vi "HEWH MW100.vi"(8 "error in":errorcluster, 11 "Message Queues out":T3) -> (0 "error out":errorcluster)   [LabVIEW 2023]
uses:
  Tenney/support/Message Queue/All Message Queues.ctl
  Tenney/support/Message Queue/Message Cluster.ctl
  Type Definitions/HEWH MW100 Data Cluster.ctl
  Custom Instrument Control/MW100/Type Definitions/HEWH Module 4 Relay Status.ctl
  Custom Instrument Control/MW100/Type Definitions/HEWH MW100 Channel Numbers.ctl
  Type Definitions/HEWH Normally Open Valve Control.ctl
  Type Definitions/HEWH Valve Bank Positions.ctl
  Type Definitions/HEWH Normally Closed Valve Control.ctl
  FVIR and LDO/support/Message Queue/Enqueue Message (Single).vi
  <vilib>/NI/Modbus Library/API/Wrapper/Create TCP Master.vi
  <vilib>/NI/Modbus Library/API/Master/Modbus Master.lvclass
  FVIR and LDO/support/Message Queue/Message Queue.lvlib
  Custom Instrument Control/MW100/Type Definitions/Station ID Selector.ctl
  Custom Instrument Control/Intellifaucet/Type Definitions/INTELLIFAUCET Set Mode.ctl
  <vilib>/NI/Modbus Library/API/Wrapper/API Main.lvlib
  Tenney/support/Message Queue/Tenney Message Queue.lvlib
panel:
  out "Loop Count":i32
  in  "Use Micro Amp Set":bool
  out "MW100 Data":T1
  in  "Pressurize Tank?":bool=TRUE
  in  "Debug":bool
  out "Debug":string[](array[string])
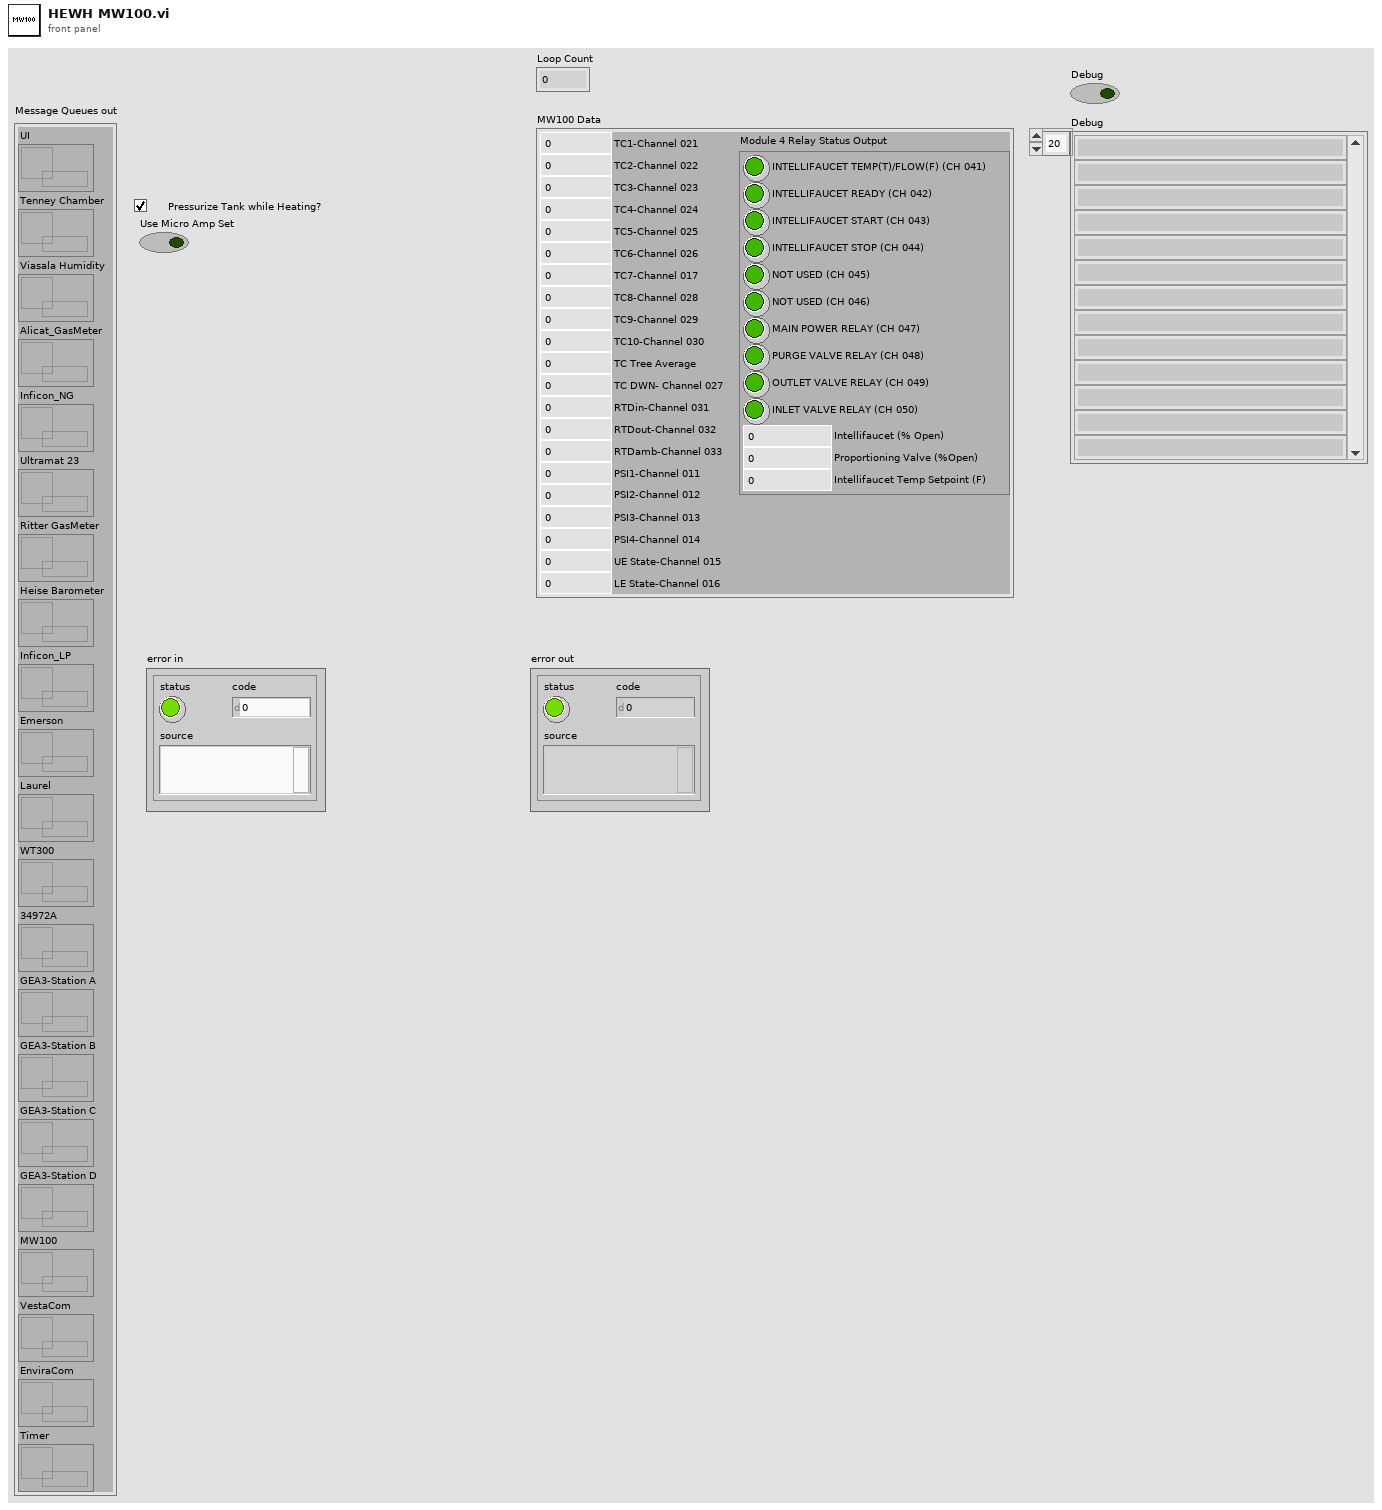
[diagram p1: front panel]
types:
  T1 = typedef "HEWH MW100 Data Cluster.ctl" = cluster{"TC1-Channel 021":dbl, "TC2-Channel 022":dbl, "TC3-Channel 023":dbl, "TC4-Channel 024":dbl, "TC5-Channel 025":dbl, "TC6-Channel 026":dbl, "TC7-Channel 017":dbl, "TC8-Channel 028":dbl, "TC9-Channel 029":dbl, "TC10-Channel 030":dbl, "TC Tree Average":dbl, "TC DWN- Channel 027":dbl, "RTDin-Channel 031":dbl, "RTDout-Channel 032":dbl, "RTDamb-Channel 033":dbl, "PSI1-Channel 011":dbl, "PSI2-Channel 012":dbl, "PSI3-Channel 013":dbl, "PSI4-Channel 014":dbl, "UE State-Channel 015":dbl, "LE State-Channel 016":dbl, "Module 4 Relay Status Output":T2}
  T2 = typedef "HEWH Module 4 Relay Status.ctl" = cluster{"INTELLIFAUCET TEMP(T)/FLOW(F) (CH 041)":bool, "INTELLIFAUCET READY (CH 042)":bool, "INTELLIFAUCET START (CH 043)":bool, "INTELLIFAUCET STOP (CH 044)":bool, "MAIN POWER RELAY (CH 047)":bool, "NOT USED (CH 045)":bool, "NOT USED (CH 046)":bool, "PURGE VALVE RELAY (CH 048)":bool, "OUTLET VALVE RELAY (CH 049)":bool, "INLET VALVE RELAY (CH 050)":bool, "Intellifaucet (% Open)":dbl, "Proportioning Valve (%Open)":dbl, "Intellifaucet Temp Setpoint (F)":dbl}
  T3 = typedef "Tenney Message Queue.lvlib/All Message Queues.ctl" = cluster{"UI":refnum<queue>, "Tenney Chamber":refnum<queue>, "Viasala Humidity":refnum<queue>, "Alicat_GasMeter":refnum<queue>, "Inficon_NG":refnum<queue>, "Ultramat 23":refnum<queue>, "Ritter GasMeter":refnum<queue>, "Heise Barometer":refnum<queue>, "Inficon_LP":refnum<queue>, "Emerson":refnum<queue>, "Laurel":refnum<queue>, "WT300":refnum<queue>, "34972A":refnum<queue>, "GEA3-Station A":refnum<queue>, "GEA3-Station B":refnum<queue>, "GEA3-Station C":refnum<queue>, "GEA3-Station D":refnum<queue>, "MW100":refnum<queue>, "VestaCom":refnum<queue>, "EnviraCom":refnum<queue>, "Timer":refnum<queue>}
  T4 = typedef "HEWH MW100 Channel Numbers.ctl" = string
  T5 = typedef "HEWH Normally Open Valve Control.ctl" = string
  T6 = typedef "HEWH Valve Bank Positions.ctl" = enum16{"Heating", "Purge", "Resting", "Draw"}
  T7 = typedef "HEWH Normally Closed Valve Control.ctl" = string
  T8 = typedef "Station ID Selector.ctl" = enum16{"", "A", "B", "C", "D", "Global"}
  T9 = typedef "INTELLIFAUCET Set Mode.ctl" = enum16{"Adjust Temp", "Adjust Flow", "Start Flow", "Stop Flow", "Hold Start", "Hold Stop", "Release Start", "Release Stop", "Temp/Flow Relay", "Adjust Prop Valve"}
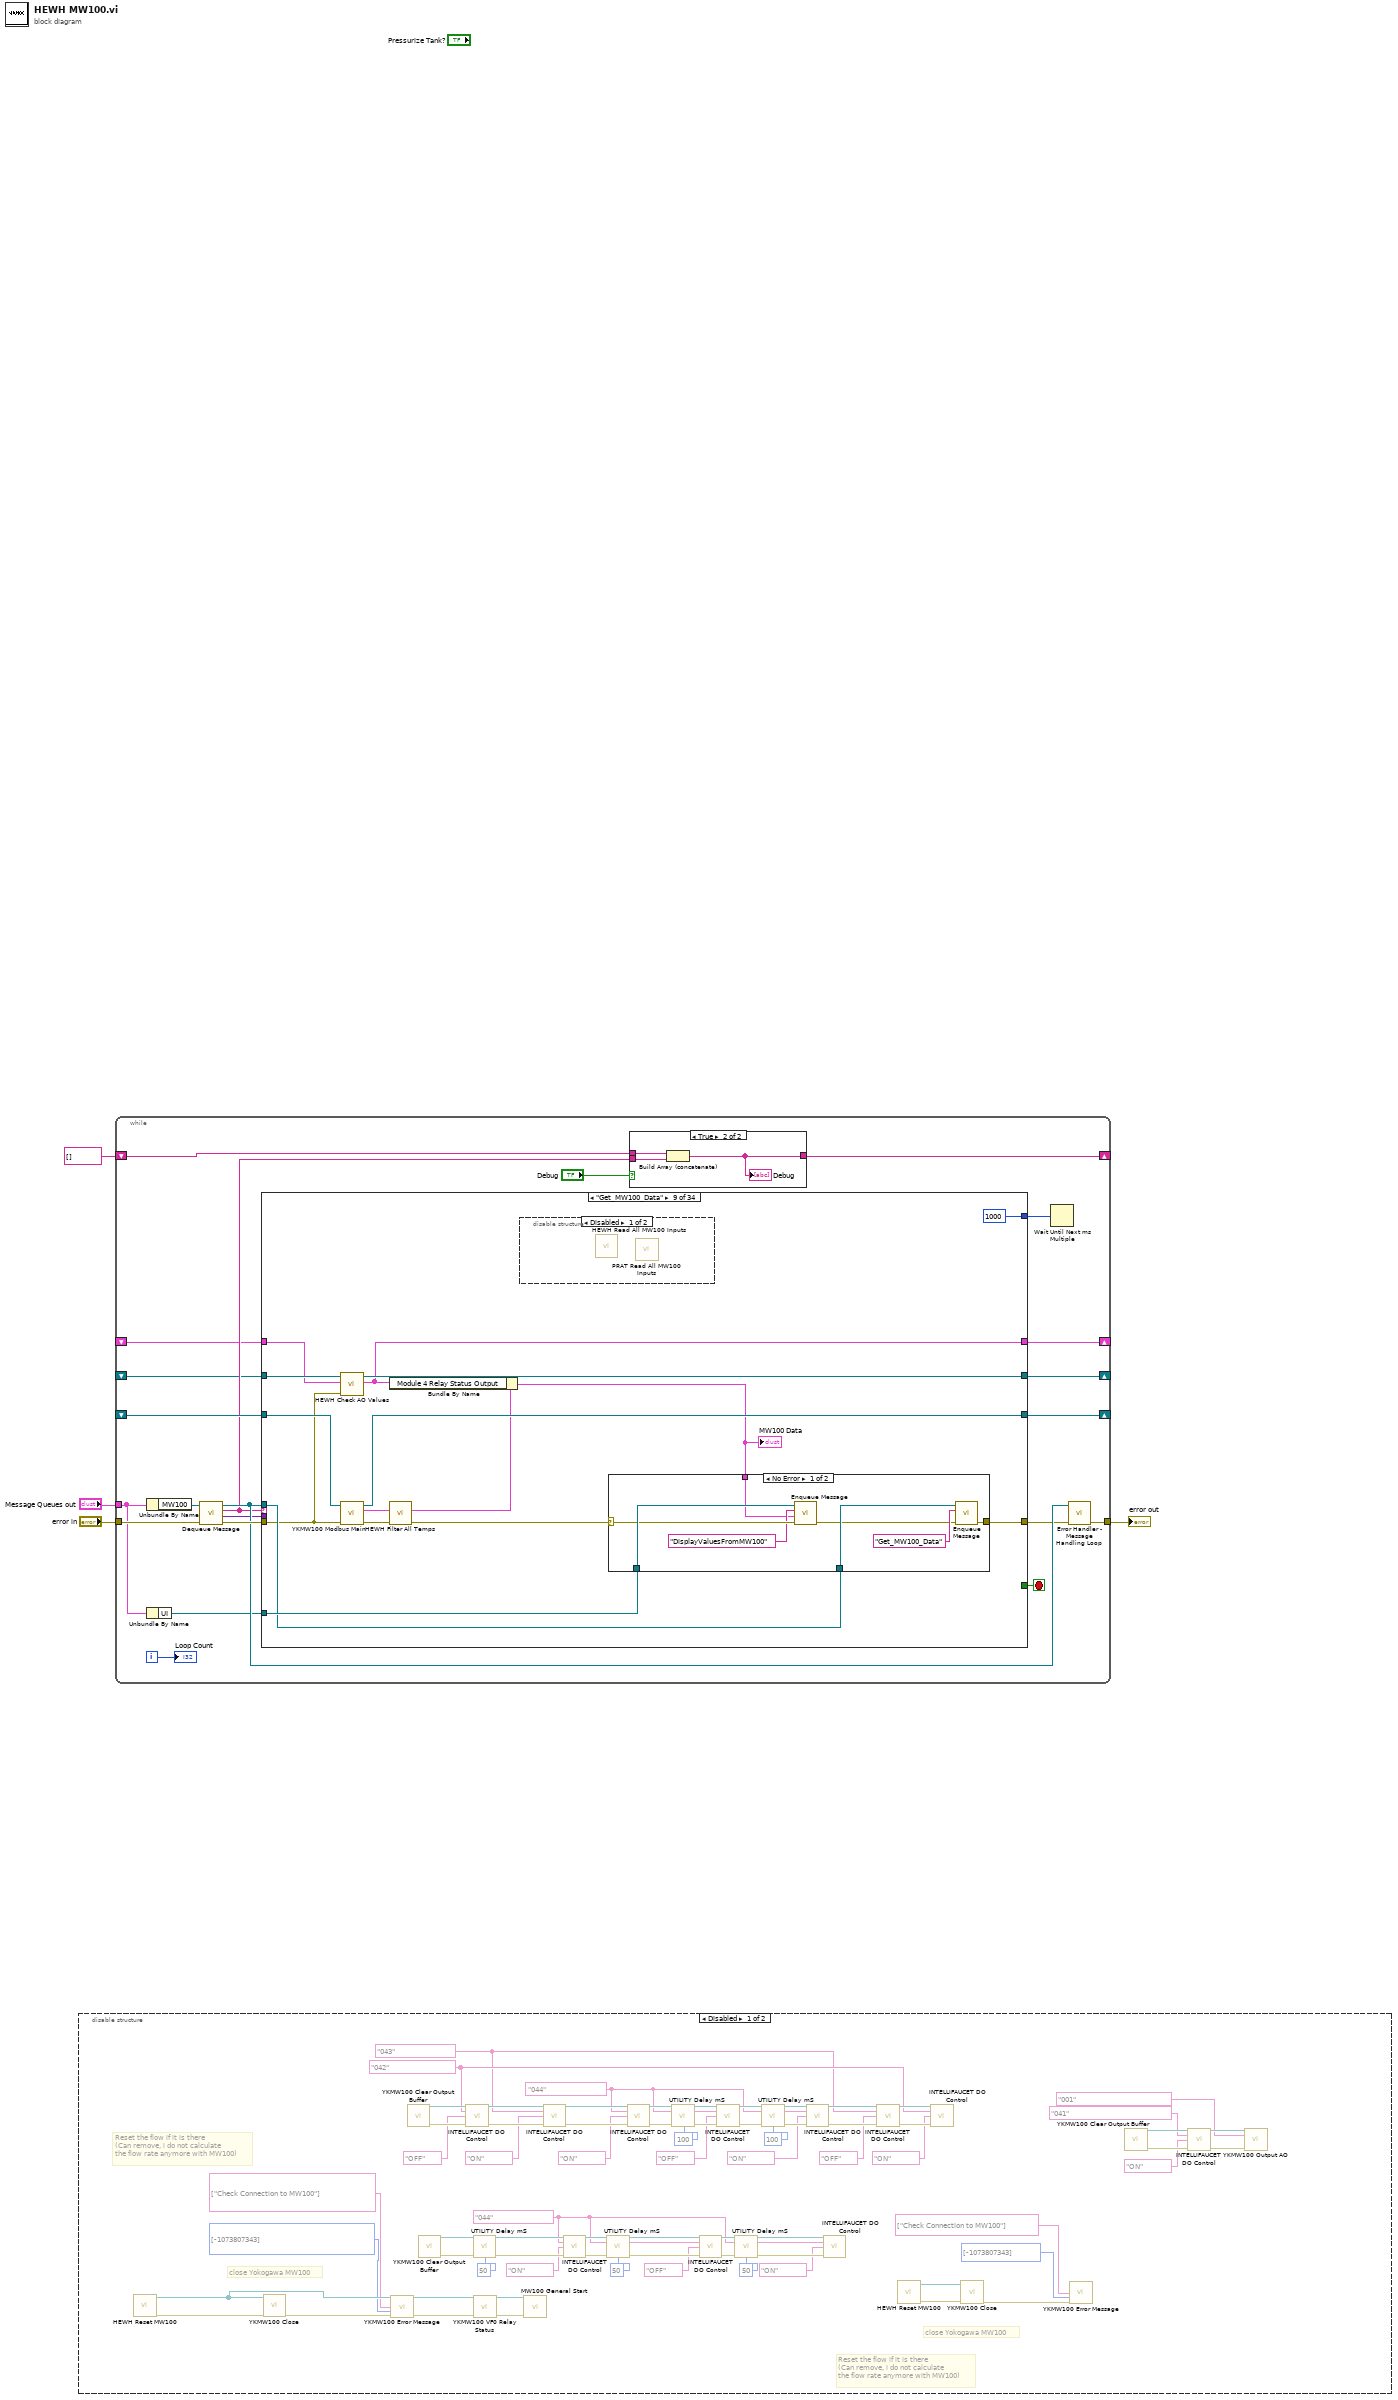
[diagram p0: block diagram]
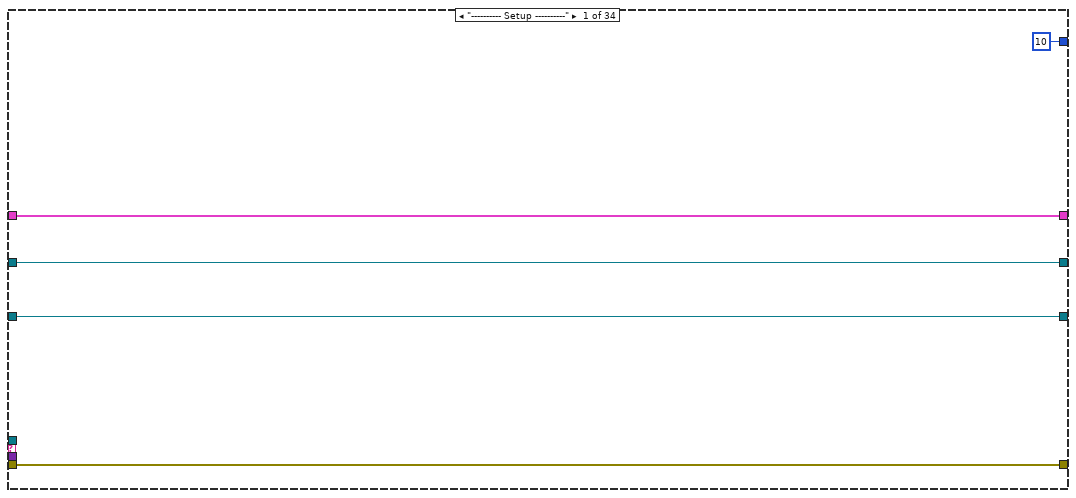
[diagram p4: hidden frame]
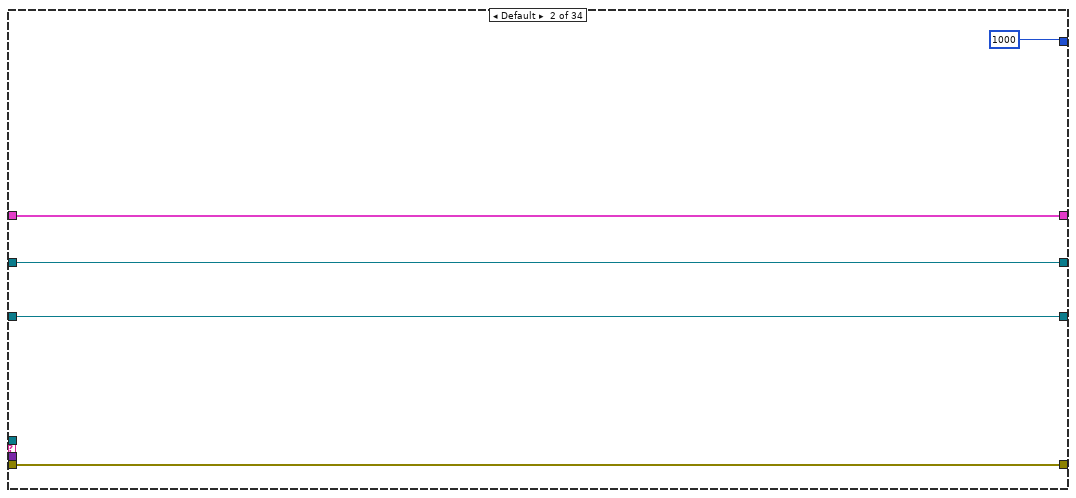
[diagram p5: hidden frame]
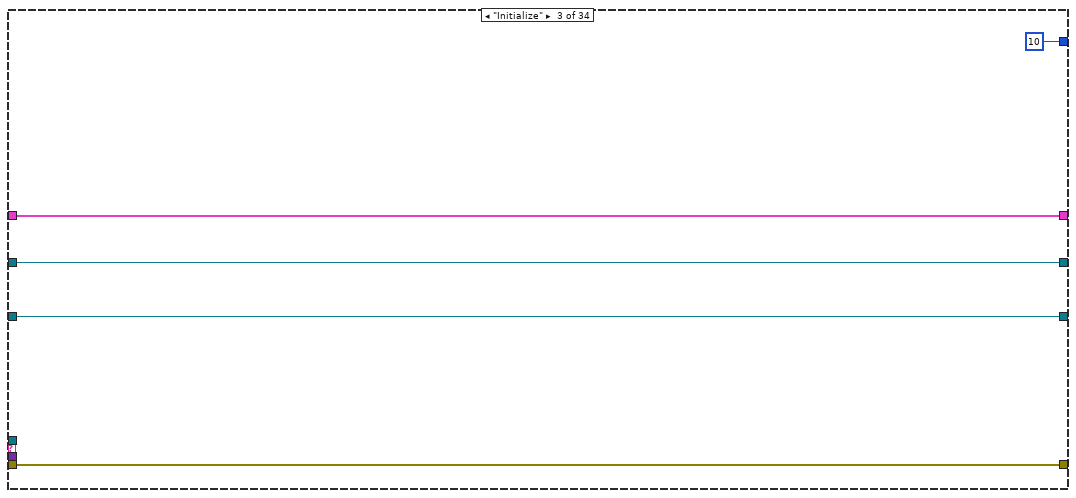
[diagram p6: hidden frame]
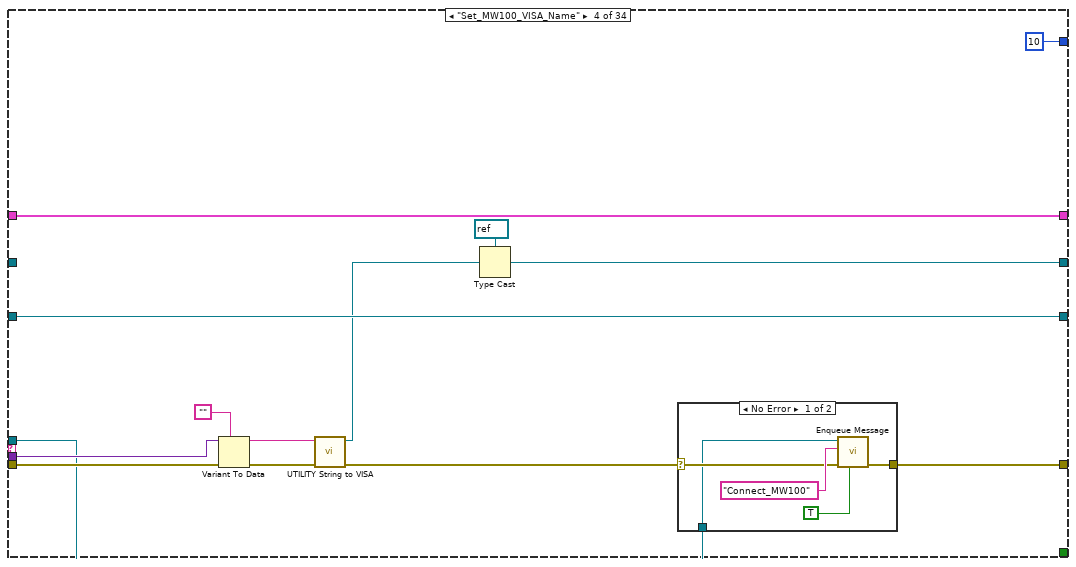
[diagram p7: hidden frame]
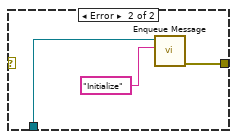
[diagram p8: hidden frame]
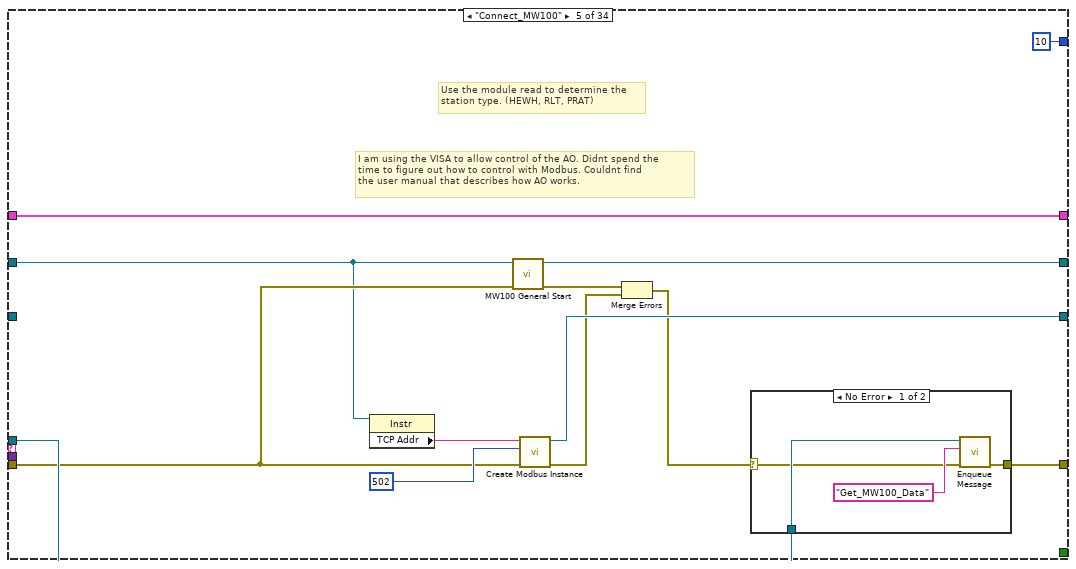
[diagram p9: hidden frame]
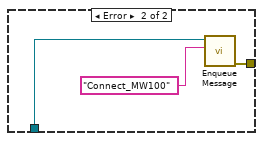
[diagram p10: hidden frame]
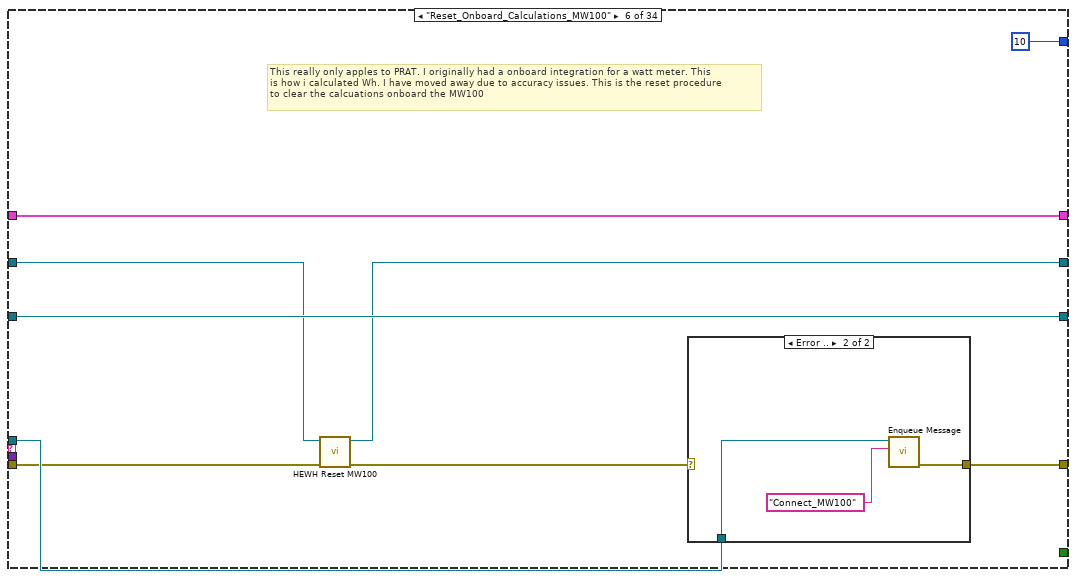
[diagram p11: hidden frame]
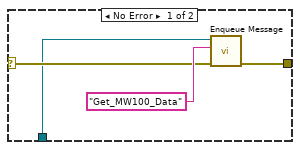
[diagram p12: hidden frame]
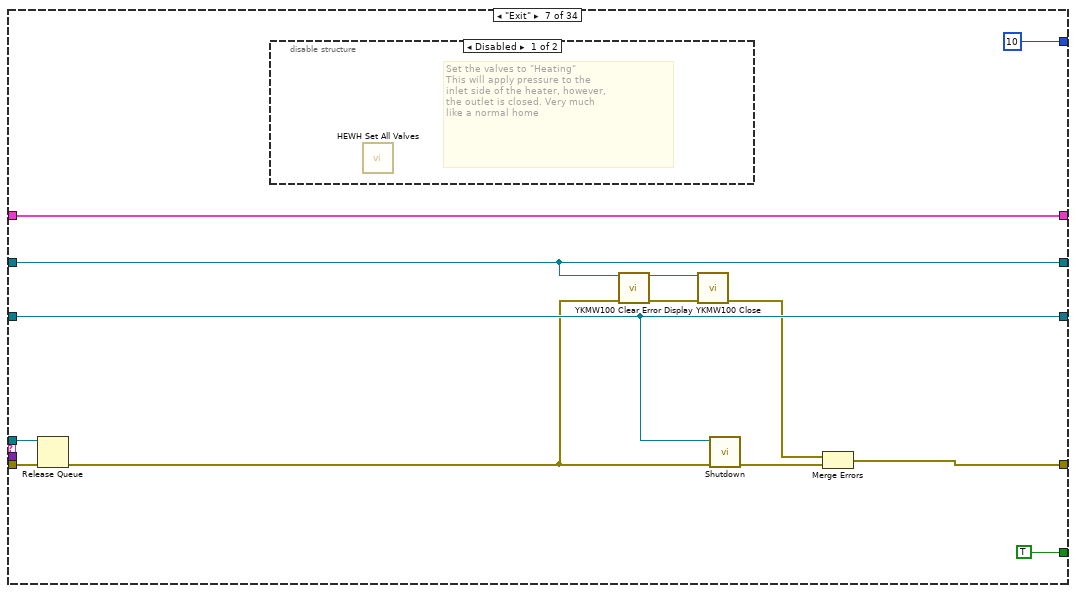
[diagram p13: hidden frame]
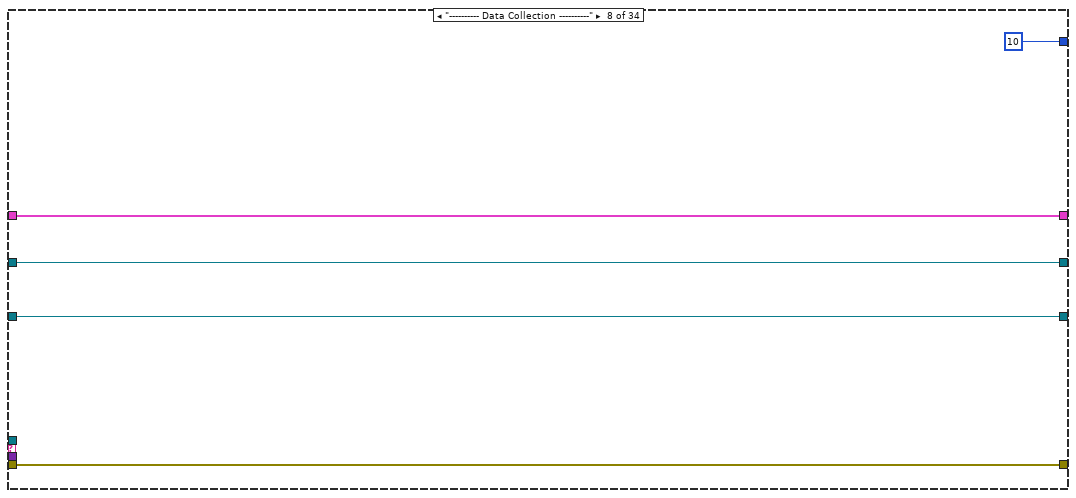
[diagram p15: hidden frame]
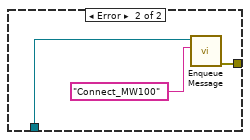
[diagram p17: hidden frame]
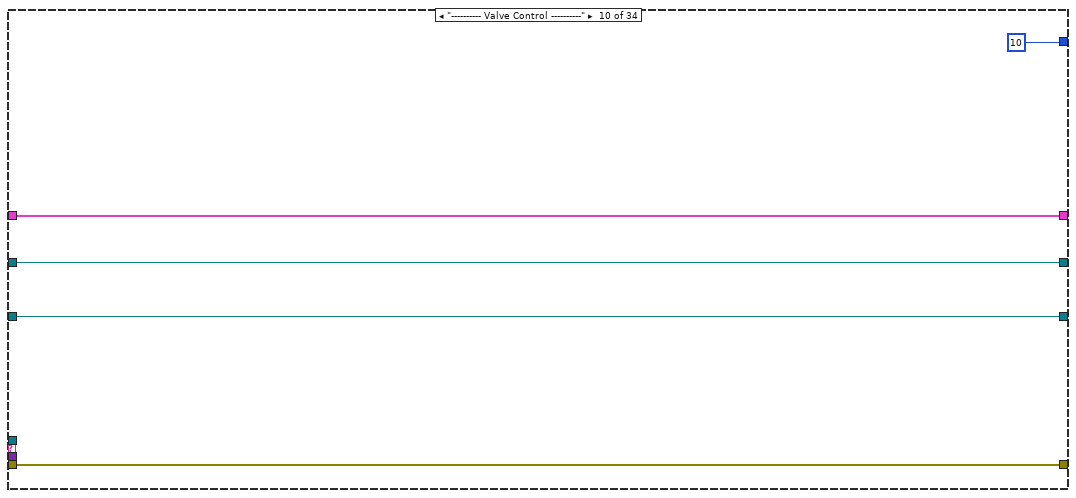
[diagram p18: hidden frame]
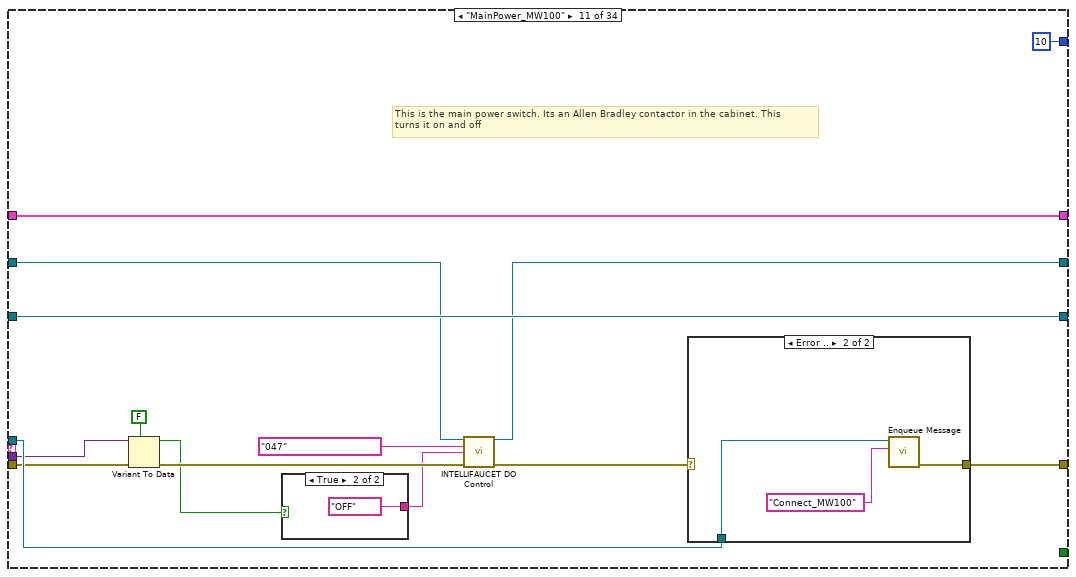
[diagram p19: hidden frame]
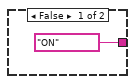
[diagram p20: hidden frame]
diagram:
  n1 = disable-structure shown="Disabled" {
    frame Disabled {
      w23 = T4 "042" ("HEWH MW100 Channel Numbers")
      w17 = T4 "043" ("HEWH MW100 Channel Numbers")
      w19 = T4 "044" ("HEWH MW100 Channel Numbers")
      w45 = T4 "044" ("HEWH MW100 Channel Numbers")
      # "Reset the flow if it is there\n(Can remove, i do not calculate\nthe flow rate anymore with MW100)"
      # "close Yokogawa MW100"
      # "Reset the flow if it is there\n(Can remove, i do not calculate\nthe flow rate anymore with MW100)"
      # "close Yokogawa MW100"
      n2 = call "HEWH Reset MW100.vi"() -> ("error out"=w64:errorcluster, "MW100 VISA Out"=w65:refnum<visa-resource-name>)  [unwired: 10 in]
      n3 = call "YKMW100 Close.vi"("VISA session"=w65, "error in (no error)"=w64) -> ("error out"=w63:errorcluster)  [unwired: 13 in]
      n4 = call "YKMW100 Error Message.vi"("VISA session"=w65, "User-Defined Descriptions"=string[] ["Check Connection to MW100"], "User-Defined Codes"=i32[] [-1073807343], "error in (no error)"=w63) -> ("dup VISA session"=w69:refnum<visa-resource-name>, "error out"=w68:errorcluster)  [unwired: 7 in, 3 out]
      n5 = call "YKMW100 Clear Output Buffer.vi"() -> ("dup VISA session"=w28:refnum<visa-resource-name>, "error out"=w29:errorcluster)  [unwired: 14 in]
      n6 = call "YKMW100 Clear Output Buffer.vi"() -> ("dup VISA session"=w52:refnum<visa-resource-name>, "error out"=w51:errorcluster)  [unwired: 14 in]
      n7 = call "INTELLIFAUCET DO Control.vi"("VISA session"=w28, "HEWH MW100 Channel Numbers"=w23, "Normally Open"=T5 "OFF", "Error In"=w29) -> ("dup VISA session"=w27:refnum<visa-resource-name>, "error out"=w26:errorcluster)  [unwired: 10 in]
      n8 = call "UTILITY Delay mS.vi"("Error In"=w51, "milliseconds to wait"=u32 50) -> ("Error Out"=w50:errorcluster)  [unwired: 13 in]
      n9 = call "YKMW100 VF0 Relay Status.vi"("MW100"=w69, "Error In"=w68) -> ("MW100 Out"=w66:refnum<visa-resource-name>, "error out"=w67:errorcluster)  [unwired: 9 in, 3 out]
      n10 = call "MW100 General Start.vi"("error in (no error)"=w67, "MW100 Input"=w66) -> ()  [unwired: 8 in, 2 out]
      n11 = call "INTELLIFAUCET DO Control.vi"("VISA session"=w27, "HEWH MW100 Channel Numbers"=w17, "Normally Open"=T5 "ON", "Error In"=w26) -> ("dup VISA session"=w35:refnum<visa-resource-name>, "error out"=w36:errorcluster)  [unwired: 10 in]
      n12 = call "INTELLIFAUCET DO Control.vi"("VISA session"=w52, "HEWH MW100 Channel Numbers"=w45, "Normally Open"=T5 "ON" ("Normally Open Valve"), "Error In"=w50) -> ("dup VISA session"=w53:refnum<visa-resource-name>, "error out"=w55:errorcluster)  [unwired: 10 in]
      n13 = call "UTILITY Delay mS.vi"("Error In"=w55, "milliseconds to wait"=u32 50) -> ("Error Out"=w54:errorcluster)  [unwired: 13 in]
      n14 = call "INTELLIFAUCET DO Control.vi"("VISA session"=w35, "HEWH MW100 Channel Numbers"=w19, "Normally Open"=T5 "ON" ("Normally Open Valve"), "Error In"=w36) -> ("dup VISA session"=w39:refnum<visa-resource-name>, "error out"=w38:errorcluster)  [unwired: 10 in]
      n15 = call "UTILITY Delay mS.vi"("Error In"=w38, "milliseconds to wait"=u32 100) -> ("Error Out"=w37:errorcluster)  [unwired: 13 in]
      n16 = call "INTELLIFAUCET DO Control.vi"("VISA session"=w53, "HEWH MW100 Channel Numbers"=w45, "Normally Open"=T5 "OFF" ("Normally Open Valve"), "Error In"=w54) -> ("dup VISA session"=w49:refnum<visa-resource-name>, "error out"=w48:errorcluster)  [unwired: 10 in]
      n17 = call "INTELLIFAUCET DO Control.vi"("VISA session"=w39, "HEWH MW100 Channel Numbers"=w19, "Normally Open"=T5 "OFF", "Error In"=w37) -> ("dup VISA session"=w33:refnum<visa-resource-name>, "error out"=w31:errorcluster)  [unwired: 10 in]
      n18 = call "UTILITY Delay mS.vi"("Error In"=w48, "milliseconds to wait"=u32 50) -> ("Error Out"=w47:errorcluster)  [unwired: 13 in]
      n19 = call "UTILITY Delay mS.vi"("Error In"=w31, "milliseconds to wait"=u32 100) -> ("Error Out"=w30:errorcluster)  [unwired: 13 in]
      n20 = call "INTELLIFAUCET DO Control.vi"("VISA session"=w33, "HEWH MW100 Channel Numbers"=w19, "Normally Open"=T5 "ON", "Error In"=w30) -> ("dup VISA session"=w32:refnum<visa-resource-name>, "error out"=w34:errorcluster)  [unwired: 10 in]
      n21 = call "INTELLIFAUCET DO Control.vi"("VISA session"=w49, "HEWH MW100 Channel Numbers"=w45, "Normally Open"=T5 "ON" ("Normally Open Valve"), "Error In"=w47) -> ()  [unwired: 10 in, 2 out]
      n22 = call "INTELLIFAUCET DO Control.vi"("VISA session"=w32, "HEWH MW100 Channel Numbers"=w17, "Normally Open"=T5 "OFF" ("Normally Open Valve"), "Error In"=w34) -> ("dup VISA session"=w25:refnum<visa-resource-name>, "error out"=w24:errorcluster)  [unwired: 10 in]
      n23 = call "HEWH Reset MW100.vi"() -> ("error out"=w59:errorcluster, "MW100 VISA Out"=w60:refnum<visa-resource-name>)  [unwired: 10 in]
      n24 = call "INTELLIFAUCET DO Control.vi"("VISA session"=w25, "HEWH MW100 Channel Numbers"=w23, "Normally Open"=T5 "ON", "Error In"=w24) -> ()  [unwired: 10 in, 2 out]
      n25 = call "YKMW100 Close.vi"("VISA session"=w60, "error in (no error)"=w59) -> ("error out"=w58:errorcluster)  [unwired: 13 in]
      n26 = call "YKMW100 Error Message.vi"("User-Defined Descriptions"=string[] ["Check Connection to MW100"], "User-Defined Codes"=i32[] [-1073807343], "error in (no error)"=w58) -> ()  [unwired: 8 in, 5 out]
      n27 = call "YKMW100 Clear Output Buffer.vi"() -> ("dup VISA session"=w10:refnum<visa-resource-name>, "error out"=w11:errorcluster)  [unwired: 14 in]
      n28 = call "INTELLIFAUCET DO Control.vi"("VISA session"=w10, "HEWH MW100 Channel Numbers"=T4 "041", "Normally Open"=T5 "ON" ("Normally Open Valve"), "Error In"=w11) -> ("dup VISA session"=w9:refnum<visa-resource-name>, "error out"=w8:errorcluster)  [unwired: 10 in]
      n29 = call "YKMW100 Output AO.vi"("VISA session"=w9, "Channel String (001)"=T4 "001" ("HEWH MW100 Channel Numbers"), "error in (no error)"=w8) -> ()  [unwired: 11 in, 2 out]
    }
    frame Enabled {
    }
  }
  n30 = while {
    tunnel: "Message Queues out" -> [w82]
    tunnel: "error in" -> [w90]
    tunnel: [w86] -> w3
    shift-right: [w84] -> _
    shift-left: _ -> [w83]
    shift-right: [w78] -> _
    shift-left: string[] [] -> [w79]
    shift-right: [w75] -> _
    shift-left: _ -> [w74]
    shift-right: [w71] -> _
    shift-left: _ -> [w70]
    i -> [w73]
    stop <- w88 stop-if-true
    n31 = Unbundle By Name(w82) -> ("MW100"=w91:refnum<queue>)
    n32 = Unbundle By Name(w82) -> ("UI"=w81:refnum<queue>)
    n33 = call "Dequeue Message.vi"("error in (no error)"=w90, "Message Queue"=w91) -> ("error out"=w89:errorcluster, "Message Data"=w76:variant, "Message"=w80:string, "dup Message Queue"=w87:refnum<queue>)  [unwired: 6 in]
    n34 = case shown="\"Get_MW100_Data\"" w80 {
      tunnel: w89 -> [w100 w103 w106 w119 w141 w157 w179 w186 w196 w218 w230 w252 w328 w404 w480 w557 w580 w604 w627 w650 w671 w692 w713 w734 w755 w776 w797 w812 w818 w835 w861 w888 w905 w923]
      tunnel: [w100 w103 w106 w121 w145 w161 w176 w186 w201 w218 w233 w255 w331 w407 w483 w560 w583 w607 w630 w653 w674 w695 w716 w737 w758 w779 w800 w812 w822 w840 w864 w890 w905 w925] -> w85
      tunnel: [_ _ _ _ _ _ TRUE _ _ _ _ _ _ _ _ _ _ _ _ _ _ _ _ _ _ _ _ _ _ _ _ _ _ _] -> w88
      tunnel: w87 -> [_ _ _ w111 w144 w160 w180 _ w200 _ w232 w254 w330 w406 w482 w559 w582 w606 w629 w652 w673 w694 w715 w736 w757 w778 w799 _ w821 w839 w863 w889 _ w924]
      tunnel: [w99 w105 w110 w124 w142 w158 w178 w185 w198 w217 w231 w253 w329 w405 w481 w558 w581 w605 w628 w651 w672 w693 w714 w735 w756 w777 w798 w811 w820 w838 w862 w886 w904 w921] -> w84
      tunnel: w83 -> [w99 w105 w110 w124 _ w158 w178 w185 w199 w217 w231 w253 w329 w405 w481 w558 w581 w605 w628 w651 w672 w693 w714 w735 w756 w777 w798 w811 w820 w838 w862 w886 w904 w921]
      tunnel: w81 -> [_ _ _ _ _ _ _ _ w202 _ _ _ _ _ _ _ _ _ _ _ _ _ _ _ _ _ _ _ _ _ _ _ _ _]
      tunnel: w76 -> [_ _ _ w116 _ _ _ _ _ _ w229 w251 w327 w403 w479 w556 w579 w603 w626 w649 w670 w691 w712 w733 w754 w775 w796 _ _ _ w860 w887 _ w922]
      tunnel: [w98 w104 w109 w112 w140 w155 w172 w184 w191 w216 w223 w245 w322 w398 w474 w551 w574 w598 w621 w647 w665 w687 w708 w728 w750 w771 w791 w810 w816 w832 w852 w880 w903 w909] -> w75
      tunnel: w74 -> [w98 w104 w109 _ w133 w156 w172 w184 w197 w216 w224 w246 w323 w399 w475 w553 w575 w599 w622 w648 w666 w688 w709 w729 w751 w772 w792 w810 w819 w833 w851 w883 w903 w915]
      tunnel: [u32 10 ("millisecond multiple") u32 1000 ("millisecond multiple") u32 10 ("millisecond multiple") u32 10 ("millisecond multiple") u32 10 ("millisecond multiple") u32 10 ("millisecond multiple") u32 10 ("millisecond multiple") u32 10 ("millisecond multiple") u32 1000 ("millisecond multiple") u32 10 ("millisecond multiple") u32 10 ("millisecond multiple") u32 10 ("millisecond multiple") u32 10 ("millisecond multiple") u32 10 ("millisecond multiple") u32 10 ("millisecond multiple") u32 10 ("millisecond multiple") u32 10 ("millisecond multiple") u32 10 ("millisecond multiple") u32 10 ("millisecond multiple") u32 10 ("millisecond multiple") u32 10 ("millisecond multiple") u32 10 ("millisecond multiple") u32 10 ("millisecond multiple") u32 10 ("millisecond multiple") u32 10 ("millisecond multiple") u32 10 ("millisecond multiple") u32 10 ("millisecond multiple") u32 10 ("millisecond multiple") u32 10 ("millisecond multiple") u32 10 ("millisecond multiple") u32 10 ("millisecond multiple") u32 10 ("millisecond multiple") u32 10 ("millisecond multiple") u32 10 ("millisecond multiple")] -> w72
      tunnel: [w96 w101 w107 w122 w134 w153 w169 w182 w188 w214 w219 w243 w319 w395 w471 w547 w570 w594 w617 w640 w661 w682 w703 w724 w745 w766 w787 w808 w813 w831 w849 w875 w901 w906] -> w71
      tunnel: w70 -> [w96 w101 w107 w122 w134 w153 w169 w182 w187 w214 w219 w243 w319 w395 w471 w547 w570 w594 w617 w640 w661 w682 w703 w724 w745 w766 w787 w808 w813 w831 w849 w875 w901 w906]
      frame "---------- Setup ----------" {
      }
      frame Default {
      }
      frame "Initialize" {
      }
      frame "Set_MW100_VISA_Name" {
        n35 = Variant To Data(error in=w119, type="", Variant=w116) -> (data=w115:string, error out=w118:errorcluster)
        n36 = call "UTILITY String to VISA.vi"("error in (no error)"=w118, "VISA Name"=w115) -> ("error out"=w117:errorcluster, "VISA resource name out"=w114:refnum<visa-resource-name>)  [unwired: 8 in]
        n37 = Type Cast(type=refnum<visa-resource-name> refnum ("dup VISA session"), x=w114) -> (*(type *) &x=w112:refnum<visa-resource-name>)
        n38 = case shown="No Error" w117 {
          selector: w117 -> [w126 _]
          tunnel: [w127 w131] -> w121
          tunnel: w111 -> [w125 w130]
          frame No Error {
            n39 = call-poly "Enqueue Message.vi"("Priority Message? (F)"=TRUE, "error in (no error)"=w126, "Message"="Connect_MW100", "Message Queue"=w125) -> ("error out"=w127:errorcluster)  [unwired: 6 in, 1 out]
          }
          frame Error {
            n40 = call-poly "Enqueue Message.vi"("Message"="Initialize", "Message Queue"=w130) -> ("error out"=w131:errorcluster)  [unwired: 8 in, 1 out]
          }
        }
      }
      frame "Connect_MW100" {
        # "Use the module read to determine the \nstation type. (HEWH, RLT, PRAT)"
        # "I am using the VISA to allow control of the AO. Didnt spend the \ntime to figure out how to control with Modbus. Couldnt find\nthe user manual that describes how AO works."
        n41 = property class="Instr"(reference=w133) -> ("TCP Addr"=w136:string)  [unwired: 1 in, 2 out]
        n42 = call "MW100 General Start.vi"("error in (no error)"=w141, "MW100 Input"=w133) -> ("error out"=w139:errorcluster, "MW100 Output"=w140:refnum<visa-resource-name>)  [unwired: 8 in]
        n43 = call-poly <vilib>:"Create Modbus Instance.vi"("error in"=w141, "port (502)"=u16 502, "address"=w136) -> ("error out"=w138:errorcluster, "TCP master instance"=w142:refnum<class "Modbus Master.lvclass">)  [unwired: 7 in]
        n44 = Merge Errors(w139, w138) -> (w137:errorcluster)
        n45 = case shown="No Error" w137 {
          selector: w137 -> [w146 _]
          tunnel: [w148 w151] -> w145
          tunnel: w144 -> [w147 w150]
          frame No Error {
            n46 = call-poly "Enqueue Message.vi"("error in (no error)"=w146, "Message"="Get_MW100_Data", "Message Queue"=w147) -> ("error out"=w148:errorcluster)  [unwired: 7 in, 1 out]
          }
          frame Error {
            n47 = call-poly "Enqueue Message.vi"("Message"="Connect_MW100", "Message Queue"=w150) -> ("error out"=w151:errorcluster)  [unwired: 8 in, 1 out]
          }
        }
      }
      frame "Reset_Onboard_Calculations_MW100" {
        # "This really only apples to PRAT. I originally had a onboard integration for a watt meter. This \nis how i calculated Wh. I have moved away due to accuracy issues. This is the reset procedure\nto clear the calcuations onboard the MW100"
        n48 = call "HEWH Reset MW100.vi"("error in (no error)"=w157, "MW100 VISA In"=w156) -> ("error out"=w159:errorcluster, "MW100 VISA Out"=w155:refnum<visa-resource-name>)  [unwired: 8 in]
        n49 = case shown="Error .." w159 {
          selector: w159 -> [w164 _]
          tunnel: [w163 w167] -> w161
          tunnel: w160 -> [w162 w166]
          frame No Error {
            n50 = call-poly "Enqueue Message.vi"("error in (no error)"=w164, "Message"="Get_MW100_Data", "Message Queue"=w162) -> ("error out"=w163:errorcluster)  [unwired: 7 in, 1 out]
          }
          frame Error {
            n51 = call-poly "Enqueue Message.vi"("Message"="Connect_MW100", "Message Queue"=w166) -> ("error out"=w167:errorcluster)  [unwired: 8 in, 1 out]
          }
        }
      }
      frame "Exit" {
        n52 = Release Queue(queue=w180, error in (no error)=w179) -> (error out=w174:errorcluster)  [unwired: 1 in, 2 out]
        n53 = disable-structure shown="Disabled" {
          frame Disabled {
            # "Set the valves to \"Heating\"\nThis will apply pressure to the\ninlet side of the heater, however,\nthe outlet is closed. Very much\nlike a normal home"
            n54 = call "HEWH Set All Valves.vi"() -> ()  [unwired: 10 in, 2 out]
          }
          frame Enabled {
          }
        }
        n55 = call "YKMW100 Clear Error Display.vi"("VISA session"=w172, "error in (no error)"=w174) -> ("dup VISA session"=w173:refnum<visa-resource-name>, "error out"=w175:errorcluster)  [unwired: 10 in, 2 out]
        n56 = call "YKMW100 Close.vi"("VISA session"=w173, "error in (no error)"=w175) -> ("error out"=w171:errorcluster)  [unwired: 13 in]
        n57 = call-dynamic "Shutdown.vi"("error in"=w174, "Modbus master in"=w178) -> ("error out"=w177:errorcluster)  [unwired: 9 in]
        n58 = Merge Errors(w171, w177) -> (w176:errorcluster)
      }
      frame "---------- Data Collection ----------" {
      }
      frame "Get_MW100_Data" {
        n59 = call "HEWH Check AO Values.vi"("error in (no error)"=w196, "Module 4 Relay Status Input"=w187, "VISA session"=w197) -> ("Module 4 Relay Status Output"=w188:T2, "dup VISA session"=w191:refnum<visa-resource-name>)  [unwired: 6 in, 1 out]
        n60 = call "YKMW100 Modbus Main.vi"("error in (no error)"=w196, "Modbus master in"=w199) -> ("error out"=w195:errorcluster, "MW Output"=w194:T1, "Modbus master out"=w198:refnum<class "Modbus Master.lvclass">)  [unwired: 7 in]
        n61 = call "HEWH Filter All Temps.vi"("error in (no error)"=w195, "Pressure Adjusted in"=w194) -> ("error out"=w189:errorcluster, "Pressure Adjusted out"=w193:T1)  [unwired: 7 in, 1 out]
        n62 = Bundle By Name(cluster=w193, "Module 4 Relay Status Output"=w188) -> (w192:T1)
        "MW100 Data" <- w192
        n63 = disable-structure shown="Disabled" {
          frame Disabled {
            n64 = call "HEWH Read All MW100 Inputs.vi"() -> ()  [unwired: 14 in, 2 out]
            n65 = call "PRAT Read All MW100 Inputs.vi"() -> ()  [unwired: 12 in, 4 out]
          }
          frame Enabled {
          }
        }
        n66 = case shown="No Error" w189 {
          selector: w189 -> [w205 _]
          tunnel: w202 -> [w210 _]
          tunnel: [w209 w212] -> w201
          tunnel: w200 -> [w208 w211]
          tunnel: w192 -> [w203 _]
          frame No Error {
            n67 = call-poly "Enqueue Message.vi"("error in (no error)"=w205, "Message Data"=w203, "Message"="DisplayValuesFromMW100", "Message Queue"=w210) -> ("error out"=w206:errorcluster)  [unwired: 6 in, 1 out]
            n68 = call-poly "Enqueue Message.vi"("error in (no error)"=w206, "Message"="Get_MW100_Data", "Message Queue"=w208) -> ("error out"=w209:errorcluster)  [unwired: 7 in, 1 out]
          }
          frame Error {
            n69 = call-poly "Enqueue Message.vi"("Message"="Connect_MW100", "Message Queue"=w211) -> ("error out"=w212:errorcluster)  [unwired: 8 in, 1 out]
          }
        }
      }
      frame "---------- Valve Control ----------" {
      }
      frame "MainPower_MW100" {
        # "This is the main power switch. Its an Allen Bradley contactor in the cabinet. This \nturns it on and off"
        n70 = Variant To Data(error in=w230, type=FALSE, Variant=w229) -> (data=w222:bool, error out=w227:errorcluster)
        n71 = case shown="True" w222 {
          tunnel: [T5 "ON" ("Normally Open Valve") T5 "OFF" ("Normally Open Valve")] -> w221
          frame False {
          }
          frame True {
          }
        }
        n72 = call "INTELLIFAUCET DO Control.vi"("VISA session"=w224, "HEWH MW100 Channel Numbers"=T4 "047", "Normally Open"=w221, "Error In"=w227) -> ("dup VISA session"=w223:refnum<visa-resource-name>, "error out"=w226:errorcluster)  [unwired: 10 in]
        n73 = case shown="Error .." w226 {
          selector: w226 -> [w238 _]
          tunnel: [w237 w241] -> w233
          tunnel: w232 -> [w236 w240]
          frame No Error {
            n74 = call-poly "Enqueue Message.vi"("error in (no error)"=w238, "Message"="Get_MW100_Data", "Message Queue"=w236) -> ("error out"=w237:errorcluster)  [unwired: 7 in, 1 out]
          }
          frame Error {
            n75 = call-poly "Enqueue Message.vi"("Message"="Connect_MW100", "Message Queue"=w240) -> ("error out"=w241:errorcluster)  [unwired: 8 in, 1 out]
          }
        }
      }
      frame "Set_Valves_StationA_MW100" {
        # "This is a function to actuate all of the valves to the proper position for heating,purge, resting, draw."
        n76 = disable-structure shown="Disabled" {
          frame Disabled {
            n77 = call "HEWH Solenoid Bank.vi"() -> ()  [unwired: 11 in, 5 out]
          }
          frame Enabled {
          }
        }
        n78 = Variant To Data(error in=w252, type=HEWH_Valve_Bank_Positions."Heating" ("Valve Bank Setting 2"), Variant=w251) -> (data=w249:T6, error out=w248:errorcluster)
        n79 = case shown="\"Heating\", Default" w249 {
          tunnel: w248 -> [w267 w279 w287 w305]
          tunnel: [w260 w274 w285 w298] -> w247
          tunnel: w246 -> [w259 w270 w284 w302]
          tunnel: [w256 w273 w286 w299] -> w245
          frame "Heating", Default {
            # "Check this one. Think its reversed."
            n80 = call "INTELLIFAUCET DO Control.vi"("VISA session"=w259, "HEWH MW100 Channel Numbers"=T4 "049", "Normally Open"=T5 "ON" ("Input Valve"), "Error In"=w267) -> ("dup VISA session"=w258:refnum<visa-resource-name>, "error out"=w264:errorcluster)  [unwired: 10 in]
            n81 = call "INTELLIFAUCET DO Control.vi"("VISA session"=w258, "HEWH MW100 Channel Numbers"=T4 "050", "Normally Open"=T5 "OFF" ("Input Valve"), "Error In"=w264) -> ("dup VISA session"=w257:refnum<visa-resource-name>, "error out"=w261:errorcluster)  [unwired: 10 in]
            n82 = call "HEWH_Normally_Closed_Solenoid.vi"("VISA session"=w257, "HEWH MW100 Channel Numbers"=T4 "048", "Normally Closed"=T7 "OFF" ("Normally Closed Valve"), "Error In"=w261) -> ("dup VISA session"=w256:refnum<visa-resource-name>, "error out"=w260:errorcluster)  [unwired: 10 in]
          }
          frame "Purge" {
            # "Check this one. Think its reversed."
            n83 = call "INTELLIFAUCET DO Control.vi"("VISA session"=w270, "HEWH MW100 Channel Numbers"=T4 "050", "Normally Open"=T5 "OFF" ("Input Valve"), "Error In"=w279) -> ("dup VISA session"=w272:refnum<visa-resource-name>, "error out"=w276:errorcluster)  [unwired: 10 in]
            n84 = call "INTELLIFAUCET DO Control.vi"("VISA session"=w272, "HEWH MW100 Channel Numbers"=T4 "049", "Normally Open"=T5 "ON" ("Input Valve"), "Error In"=w276) -> ("dup VISA session"=w271:refnum<visa-resource-name>, "error out"=w275:errorcluster)  [unwired: 10 in]
            n85 = call "HEWH_Normally_Closed_Solenoid.vi"("VISA session"=w271, "HEWH MW100 Channel Numbers"=T4 "048", "Normally Closed"=T7 "ON" ("Normally Closed Valve"), "Error In"=w275) -> ("dup VISA session"=w273:refnum<visa-resource-name>, "error out"=w274:errorcluster)  [unwired: 10 in]
          }
          frame "Resting" {
            # "Check this one. Think its reversed."
            n86 = call "INTELLIFAUCET DO Control.vi"("VISA session"=w284, "HEWH MW100 Channel Numbers"=T4 "050", "Normally Open"=T5 "ON" ("Input Valve"), "Error In"=w287) -> ("dup VISA session"=w295:refnum<visa-resource-name>, "error out"=w297:errorcluster)  [unwired: 10 in]
            n87 = call "INTELLIFAUCET DO Control.vi"("VISA session"=w295, "HEWH MW100 Channel Numbers"=T4 "049", "Normally Open"=T5 "OFF" ("Input Valve"), "Error In"=w297) -> ("dup VISA session"=w294:refnum<visa-resource-name>, "error out"=w296:errorcluster)  [unwired: 10 in]
            n88 = call "HEWH_Normally_Closed_Solenoid.vi"("VISA session"=w294, "HEWH MW100 Channel Numbers"=T4 "048", "Normally Closed"=T7 "OFF" ("Normally Closed Valve"), "Error In"=w296) -> ("dup VISA session"=w286:refnum<visa-resource-name>, "error out"=w285:errorcluster)  [unwired: 10 in]
          }
          frame "Draw" {
            # "Check this one. Think its reversed."
            n89 = call "HEWH_Normally_Closed_Solenoid.vi"("VISA session"=w302, "HEWH MW100 Channel Numbers"=T4 "048", "Normally Closed"=T7 "OFF" ("Normally Closed Valve"), "Error In"=w305) -> ("dup VISA session"=w301:refnum<visa-resource-name>, "error out"=w304:errorcluster)  [unwired: 10 in]
            n90 = call "INTELLIFAUCET DO Control.vi"("VISA session"=w301, "HEWH MW100 Channel Numbers"=T4 "050", "Normally Open"=T5 "OFF" ("Input Valve"), "Error In"=w304) -> ("dup VISA session"=w300:refnum<visa-resource-name>, "error out"=w303:errorcluster)  [unwired: 10 in]
            n91 = call "INTELLIFAUCET DO Control.vi"("VISA session"=w300, "HEWH MW100 Channel Numbers"=T4 "049", "Normally Open"=T5 "OFF" ("Input Valve"), "Error In"=w303) -> ("dup VISA session"=w299:refnum<visa-resource-name>, "error out"=w298:errorcluster)  [unwired: 10 in]
          }
        }
        n92 = case shown="Error .." w247 {
          selector: w247 -> [w314 _]
          tunnel: [w313 w317] -> w255
          tunnel: w254 -> [w312 w316]
          frame No Error {
            n93 = call-poly "Enqueue Message.vi"("error in (no error)"=w314, "Message"="Get_MW100_Data", "Message Queue"=w312) -> ("error out"=w313:errorcluster)  [unwired: 7 in, 1 out]
          }
          frame Error {
            n94 = call-poly "Enqueue Message.vi"("Message"="Connect_MW100", "Message Queue"=w316) -> ("error out"=w317:errorcluster)  [unwired: 8 in, 1 out]
          }
        }
      }
      frame "Set_Valves_StationB_MW100" {
        # "This is a function to actuate all of the valves to the proper position for heating,purge, resting, draw."
        n95 = Variant To Data(error in=w328, type=HEWH_Valve_Bank_Positions."Heating" ("Valve Bank Setting 2"), Variant=w327) -> (data=w324:T6, error out=w325:errorcluster)
        n96 = case shown="\"Draw\"" w324 {
          tunnel: w325 -> [w343 w355 w363 w381]
          tunnel: [w336 w350 w361 w374] -> w321
          tunnel: w323 -> [w335 w346 w360 w378]
          tunnel: [w332 w349 w362 w375] -> w322
          frame "Heating", Default {
            # "Check this one. Think its reversed."
            n97 = call "INTELLIFAUCET DO Control.vi"("VISA session"=w335, "HEWH MW100 Channel Numbers"=T4 "052", "Normally Open"=T5 "ON" ("Input Valve"), "Error In"=w343) -> ("dup VISA session"=w334:refnum<visa-resource-name>, "error out"=w340:errorcluster)  [unwired: 10 in]
            n98 = call "INTELLIFAUCET DO Control.vi"("VISA session"=w334, "HEWH MW100 Channel Numbers"=T4 "053", "Normally Open"=T5 "OFF" ("Input Valve"), "Error In"=w340) -> ("dup VISA session"=w333:refnum<visa-resource-name>, "error out"=w337:errorcluster)  [unwired: 10 in]
            n99 = call "HEWH_Normally_Closed_Solenoid.vi"("VISA session"=w333, "HEWH MW100 Channel Numbers"=T4 "051", "Normally Closed"=T7 "OFF" ("Normally Closed Valve"), "Error In"=w337) -> ("dup VISA session"=w332:refnum<visa-resource-name>, "error out"=w336:errorcluster)  [unwired: 10 in]
          }
          frame "Purge" {
            # "Check this one. Think its reversed."
            n100 = call "INTELLIFAUCET DO Control.vi"("VISA session"=w346, "HEWH MW100 Channel Numbers"=T4 "053", "Normally Open"=T5 "OFF" ("Input Valve"), "Error In"=w355) -> ("dup VISA session"=w348:refnum<visa-resource-name>, "error out"=w352:errorcluster)  [unwired: 10 in]
            n101 = call "INTELLIFAUCET DO Control.vi"("VISA session"=w348, "HEWH MW100 Channel Numbers"=T4 "052", "Normally Open"=T5 "ON" ("Input Valve"), "Error In"=w352) -> ("dup VISA session"=w347:refnum<visa-resource-name>, "error out"=w351:errorcluster)  [unwired: 10 in]
            n102 = call "HEWH_Normally_Closed_Solenoid.vi"("VISA session"=w347, "HEWH MW100 Channel Numbers"=T4 "051", "Normally Closed"=T7 "ON" ("Normally Closed Valve"), "Error In"=w351) -> ("dup VISA session"=w349:refnum<visa-resource-name>, "error out"=w350:errorcluster)  [unwired: 10 in]
          }
          frame "Resting" {
            # "Check this one. Think its reversed."
            n103 = call "INTELLIFAUCET DO Control.vi"("VISA session"=w360, "HEWH MW100 Channel Numbers"=T4 "053", "Normally Open"=T5 "ON" ("Input Valve"), "Error In"=w363) -> ("dup VISA session"=w371:refnum<visa-resource-name>, "error out"=w373:errorcluster)  [unwired: 10 in]
            n104 = call "INTELLIFAUCET DO Control.vi"("VISA session"=w371, "HEWH MW100 Channel Numbers"=T4 "052", "Normally Open"=T5 "OFF" ("Input Valve"), "Error In"=w373) -> ("dup VISA session"=w370:refnum<visa-resource-name>, "error out"=w372:errorcluster)  [unwired: 10 in]
            n105 = call "HEWH_Normally_Closed_Solenoid.vi"("VISA session"=w370, "HEWH MW100 Channel Numbers"=T4 "051", "Normally Closed"=T7 "OFF" ("Normally Closed Valve"), "Error In"=w372) -> ("dup VISA session"=w362:refnum<visa-resource-name>, "error out"=w361:errorcluster)  [unwired: 10 in]
          }
          frame "Draw" {
            # "Check this one. Think its reversed."
            n106 = call "HEWH_Normally_Closed_Solenoid.vi"("VISA session"=w378, "HEWH MW100 Channel Numbers"=T4 "051", "Normally Closed"=T7 "OFF" ("Normally Closed Valve"), "Error In"=w381) -> ("dup VISA session"=w377:refnum<visa-resource-name>, "error out"=w380:errorcluster)  [unwired: 10 in]
            n107 = call "INTELLIFAUCET DO Control.vi"("VISA session"=w377, "HEWH MW100 Channel Numbers"=T4 "053", "Normally Open"=T5 "OFF" ("Input Valve"), "Error In"=w380) -> ("dup VISA session"=w376:refnum<visa-resource-name>, "error out"=w379:errorcluster)  [unwired: 10 in]
            n108 = call "INTELLIFAUCET DO Control.vi"("VISA session"=w376, "HEWH MW100 Channel Numbers"=T4 "052", "Normally Open"=T5 "OFF" ("Input Valve"), "Error In"=w379) -> ("dup VISA session"=w375:refnum<visa-resource-name>, "error out"=w374:errorcluster)  [unwired: 10 in]
          }
        }
        n109 = disable-structure shown="Disabled" {
          frame Disabled {
            n110 = call "HEWH Solenoid Bank.vi"() -> ()  [unwired: 11 in, 5 out]
          }
          frame Enabled {
          }
        }
        n111 = case shown="Error .." w321 {
          selector: w321 -> [w390 _]
          tunnel: [w389 w393] -> w331
          tunnel: w330 -> [w388 w392]
          frame No Error {
            n112 = call-poly "Enqueue Message.vi"("error in (no error)"=w390, "Message"="Get_MW100_Data", "Message Queue"=w388) -> ("error out"=w389:errorcluster)  [unwired: 7 in, 1 out]
          }
          frame Error {
            n113 = call-poly "Enqueue Message.vi"("Message"="Connect_MW100", "Message Queue"=w392) -> ("error out"=w393:errorcluster)  [unwired: 8 in, 1 out]
          }
        }
      }
      frame "Set_Valves_StationC_MW100" {
        # "This is a function to actuate all of the valves to the proper position for heating,purge, resting, draw."
        n114 = Variant To Data(error in=w404, type=HEWH_Valve_Bank_Positions."Heating" ("Valve Bank Setting 2"), Variant=w403) -> (data=w400:T6, error out=w401:errorcluster)
        n115 = case shown="\"Draw\"" w400 {
          tunnel: w401 -> [w419 w431 w439 w457]
          tunnel: [w412 w426 w437 w450] -> w397
          tunnel: w399 -> [w411 w422 w436 w454]
          tunnel: [w408 w425 w438 w451] -> w398
          frame "Heating", Default {
            # "Check this one. Think its reversed."
            n116 = call "INTELLIFAUCET DO Control.vi"("VISA session"=w411, "HEWH MW100 Channel Numbers"=T4 "055", "Normally Open"=T5 "ON" ("Input Valve"), "Error In"=w419) -> ("dup VISA session"=w410:refnum<visa-resource-name>, "error out"=w416:errorcluster)  [unwired: 10 in]
            n117 = call "INTELLIFAUCET DO Control.vi"("VISA session"=w410, "HEWH MW100 Channel Numbers"=T4 "057", "Normally Open"=T5 "OFF" ("Input Valve"), "Error In"=w416) -> ("dup VISA session"=w409:refnum<visa-resource-name>, "error out"=w413:errorcluster)  [unwired: 10 in]
            n118 = call "HEWH_Normally_Closed_Solenoid.vi"("VISA session"=w409, "HEWH MW100 Channel Numbers"=T4 "054", "Normally Closed"=T7 "OFF" ("Normally Closed Valve"), "Error In"=w413) -> ("dup VISA session"=w408:refnum<visa-resource-name>, "error out"=w412:errorcluster)  [unwired: 10 in]
          }
          frame "Purge" {
            # "Check this one. Think its reversed."
            n119 = call "INTELLIFAUCET DO Control.vi"("VISA session"=w422, "HEWH MW100 Channel Numbers"=T4 "057", "Normally Open"=T5 "OFF" ("Input Valve"), "Error In"=w431) -> ("dup VISA session"=w424:refnum<visa-resource-name>, "error out"=w428:errorcluster)  [unwired: 10 in]
            n120 = call "INTELLIFAUCET DO Control.vi"("VISA session"=w424, "HEWH MW100 Channel Numbers"=T4 "055", "Normally Open"=T5 "ON" ("Input Valve"), "Error In"=w428) -> ("dup VISA session"=w423:refnum<visa-resource-name>, "error out"=w427:errorcluster)  [unwired: 10 in]
            n121 = call "HEWH_Normally_Closed_Solenoid.vi"("VISA session"=w423, "HEWH MW100 Channel Numbers"=T4 "054", "Normally Closed"=T7 "ON" ("Normally Closed Valve"), "Error In"=w427) -> ("dup VISA session"=w425:refnum<visa-resource-name>, "error out"=w426:errorcluster)  [unwired: 10 in]
          }
          frame "Resting" {
            # "Check this one. Think its reversed."
            n122 = call "INTELLIFAUCET DO Control.vi"("VISA session"=w436, "HEWH MW100 Channel Numbers"=T4 "057", "Normally Open"=T5 "ON" ("Input Valve"), "Error In"=w439) -> ("dup VISA session"=w447:refnum<visa-resource-name>, "error out"=w449:errorcluster)  [unwired: 10 in]
            n123 = call "INTELLIFAUCET DO Control.vi"("VISA session"=w447, "HEWH MW100 Channel Numbers"=T4 "055", "Normally Open"=T5 "OFF" ("Input Valve"), "Error In"=w449) -> ("dup VISA session"=w446:refnum<visa-resource-name>, "error out"=w448:errorcluster)  [unwired: 10 in]
            n124 = call "HEWH_Normally_Closed_Solenoid.vi"("VISA session"=w446, "HEWH MW100 Channel Numbers"=T4 "054", "Normally Closed"=T7 "OFF" ("Normally Closed Valve"), "Error In"=w448) -> ("dup VISA session"=w438:refnum<visa-resource-name>, "error out"=w437:errorcluster)  [unwired: 10 in]
          }
          frame "Draw" {
            # "Check this one. Think its reversed."
            n125 = call "HEWH_Normally_Closed_Solenoid.vi"("VISA session"=w454, "HEWH MW100 Channel Numbers"=T4 "054", "Normally Closed"=T7 "OFF" ("Normally Closed Valve"), "Error In"=w457) -> ("dup VISA session"=w453:refnum<visa-resource-name>, "error out"=w456:errorcluster)  [unwired: 10 in]
            n126 = call "INTELLIFAUCET DO Control.vi"("VISA session"=w453, "HEWH MW100 Channel Numbers"=T4 "057", "Normally Open"=T5 "OFF" ("Input Valve"), "Error In"=w456) -> ("dup VISA session"=w452:refnum<visa-resource-name>, "error out"=w455:errorcluster)  [unwired: 10 in]
            n127 = call "INTELLIFAUCET DO Control.vi"("VISA session"=w452, "HEWH MW100 Channel Numbers"=T4 "055", "Normally Open"=T5 "OFF" ("Input Valve"), "Error In"=w455) -> ("dup VISA session"=w451:refnum<visa-resource-name>, "error out"=w450:errorcluster)  [unwired: 10 in]
          }
        }
        n128 = disable-structure shown="Disabled" {
          frame Disabled {
            n129 = call "HEWH Solenoid Bank.vi"() -> ()  [unwired: 11 in, 5 out]
          }
          frame Enabled {
          }
        }
        n130 = case shown="Error .." w397 {
          selector: w397 -> [w466 _]
          tunnel: [w465 w469] -> w407
          tunnel: w406 -> [w464 w468]
          frame No Error {
            n131 = call-poly "Enqueue Message.vi"("error in (no error)"=w466, "Message"="Get_MW100_Data", "Message Queue"=w464) -> ("error out"=w465:errorcluster)  [unwired: 7 in, 1 out]
          }
          frame Error {
            n132 = call-poly "Enqueue Message.vi"("Message"="Connect_MW100", "Message Queue"=w468) -> ("error out"=w469:errorcluster)  [unwired: 8 in, 1 out]
          }
        }
      }
      frame "Set_Valves_StationD_MW100" {
        # "This is a function to actuate all of the valves to the proper position for heating,purge, resting, draw."
        n133 = Variant To Data(error in=w480, type=HEWH_Valve_Bank_Positions."Heating" ("Valve Bank Setting 2"), Variant=w479) -> (data=w476:T6, error out=w477:errorcluster)
        n134 = case shown="\"Heating\", Default" w476 {
          tunnel: w477 -> [w495 w507 w515 w533]
          tunnel: [w488 w502 w513 w526] -> w473
          tunnel: w475 -> [w487 w498 w512 w530]
          tunnel: [w484 w501 w514 w527] -> w474
          frame "Heating", Default {
            # "Check this one. Think its reversed."
            n135 = call "INTELLIFAUCET DO Control.vi"("VISA session"=w487, "HEWH MW100 Channel Numbers"=T4 "059", "Normally Open"=T5 "ON" ("Input Valve"), "Error In"=w495) -> ("dup VISA session"=w486:refnum<visa-resource-name>, "error out"=w492:errorcluster)  [unwired: 10 in]
            n136 = call "INTELLIFAUCET DO Control.vi"("VISA session"=w486, "HEWH MW100 Channel Numbers"=T4 "060", "Normally Open"=T5 "OFF" ("Input Valve"), "Error In"=w492) -> ("dup VISA session"=w485:refnum<visa-resource-name>, "error out"=w489:errorcluster)  [unwired: 10 in]
            n137 = call "HEWH_Normally_Closed_Solenoid.vi"("VISA session"=w485, "HEWH MW100 Channel Numbers"=T4 "058", "Normally Closed"=T7 "OFF" ("Normally Closed Valve"), "Error In"=w489) -> ("dup VISA session"=w484:refnum<visa-resource-name>, "error out"=w488:errorcluster)  [unwired: 10 in]
          }
          frame "Purge" {
            # "Check this one. Think its reversed."
            n138 = call "INTELLIFAUCET DO Control.vi"("VISA session"=w498, "HEWH MW100 Channel Numbers"=T4 "060", "Normally Open"=T5 "OFF" ("Input Valve"), "Error In"=w507) -> ("dup VISA session"=w500:refnum<visa-resource-name>, "error out"=w504:errorcluster)  [unwired: 10 in]
            n139 = call "INTELLIFAUCET DO Control.vi"("VISA session"=w500, "HEWH MW100 Channel Numbers"=T4 "059", "Normally Open"=T5 "ON" ("Input Valve"), "Error In"=w504) -> ("dup VISA session"=w499:refnum<visa-resource-name>, "error out"=w503:errorcluster)  [unwired: 10 in]
            n140 = call "HEWH_Normally_Closed_Solenoid.vi"("VISA session"=w499, "HEWH MW100 Channel Numbers"=T4 "058", "Normally Closed"=T7 "ON" ("Normally Closed Valve"), "Error In"=w503) -> ("dup VISA session"=w501:refnum<visa-resource-name>, "error out"=w502:errorcluster)  [unwired: 10 in]
          }
          frame "Resting" {
            # "Check this one. Think its reversed."
            n141 = call "INTELLIFAUCET DO Control.vi"("VISA session"=w512, "HEWH MW100 Channel Numbers"=T4 "060", "Normally Open"=T5 "ON" ("Input Valve"), "Error In"=w515) -> ("dup VISA session"=w523:refnum<visa-resource-name>, "error out"=w525:errorcluster)  [unwired: 10 in]
            n142 = call "INTELLIFAUCET DO Control.vi"("VISA session"=w523, "HEWH MW100 Channel Numbers"=T4 "059", "Normally Open"=T5 "OFF" ("Input Valve"), "Error In"=w525) -> ("dup VISA session"=w522:refnum<visa-resource-name>, "error out"=w524:errorcluster)  [unwired: 10 in]
            n143 = call "HEWH_Normally_Closed_Solenoid.vi"("VISA session"=w522, "HEWH MW100 Channel Numbers"=T4 "058", "Normally Closed"=T7 "OFF" ("Normally Closed Valve"), "Error In"=w524) -> ("dup VISA session"=w514:refnum<visa-resource-name>, "error out"=w513:errorcluster)  [unwired: 10 in]
          }
          frame "Draw" {
            # "Check this one. Think its reversed."
            n144 = call "HEWH_Normally_Closed_Solenoid.vi"("VISA session"=w530, "HEWH MW100 Channel Numbers"=T4 "058", "Normally Closed"=T7 "OFF" ("Normally Closed Valve"), "Error In"=w533) -> ("dup VISA session"=w529:refnum<visa-resource-name>, "error out"=w532:errorcluster)  [unwired: 10 in]
            n145 = call "INTELLIFAUCET DO Control.vi"("VISA session"=w529, "HEWH MW100 Channel Numbers"=T4 "060", "Normally Open"=T5 "OFF" ("Input Valve"), "Error In"=w532) -> ("dup VISA session"=w528:refnum<visa-resource-name>, "error out"=w531:errorcluster)  [unwired: 10 in]
            n146 = call "INTELLIFAUCET DO Control.vi"("VISA session"=w528, "HEWH MW100 Channel Numbers"=T4 "059", "Normally Open"=T5 "OFF" ("Input Valve"), "Error In"=w531) -> ("dup VISA session"=w527:refnum<visa-resource-name>, "error out"=w526:errorcluster)  [unwired: 10 in]
          }
        }
        n147 = disable-structure shown="Disabled" {
          frame Disabled {
            n148 = call "HEWH Solenoid Bank.vi"() -> ()  [unwired: 11 in, 5 out]
          }
          frame Enabled {
          }
        }
        n149 = case shown="Error .." w473 {
          selector: w473 -> [w542 _]
          tunnel: [w541 w545] -> w483
          tunnel: w482 -> [w540 w544]
          frame No Error {
            n150 = call-poly "Enqueue Message.vi"("error in (no error)"=w542, "Message"="Get_MW100_Data", "Message Queue"=w540) -> ("error out"=w541:errorcluster)  [unwired: 7 in, 1 out]
          }
          frame Error {
            n151 = call-poly "Enqueue Message.vi"("Message"="Connect_MW100", "Message Queue"=w544) -> ("error out"=w545:errorcluster)  [unwired: 8 in, 1 out]
          }
        }
      }
      frame "Inlet_Valve_A_MW100" {
        # "Check this one. Think its reversed."
        n152 = disable-structure shown="Disabled" {
          frame Disabled {
            n153 = call "Solenoid - Fill.vi"() -> ()  [unwired: 10 in, 2 out]
            n154 = call "HEWH PRAT Valves.vi"("Normally Closed Valve?"=TRUE, "Station ID"=Station_ID_Selector."A") -> ()  [unwired: 7 in, 3 out]
          }
          frame Enabled {
          }
        }
        n155 = Variant To Data(error in=w557, type=T5 "ON" ("Input Valve"), Variant=w556) -> (data=w549:T5, error out=w555:errorcluster)
        n156 = call "INTELLIFAUCET DO Control.vi"("VISA session"=w553, "HEWH MW100 Channel Numbers"=T4 "050", "Normally Open"=w549, "Error In"=w555) -> ("dup VISA session"=w551:refnum<visa-resource-name>, "error out"=w552:errorcluster)  [unwired: 10 in]
        n157 = case shown="Error .." w552 {
          selector: w552 -> [w565 _]
          tunnel: [w564 w568] -> w560
          tunnel: w559 -> [w563 w567]
          frame No Error {
            n158 = call-poly "Enqueue Message.vi"("error in (no error)"=w565, "Message"="Get_MW100_Data", "Message Queue"=w563) -> ("error out"=w564:errorcluster)  [unwired: 7 in, 1 out]
          }
          frame Error {
            n159 = call-poly "Enqueue Message.vi"("Message"="Connect_MW100", "Message Queue"=w567) -> ("error out"=w568:errorcluster)  [unwired: 8 in, 1 out]
          }
        }
      }
      frame "Inlet_Valve_B_MW100" {
        # "Check this one. Think its reversed."
        n160 = Variant To Data(error in=w580, type=T5 "ON" ("Input Valve"), Variant=w579) -> (data=w572:T5, error out=w576:errorcluster)
        n161 = disable-structure shown="Disabled" {
          frame Disabled {
            n162 = case shown="\"PRAT\"" {
              selector: _ -> [_ _]
              tunnel: [_ w586] -> _
              frame Default {
                n163 = call "Solenoid - Fill.vi"() -> ()  [unwired: 10 in, 2 out]
              }
              frame "PRAT" {
                n164 = call "HEWH PRAT Valves.vi"("Normally Closed Valve?"=TRUE, "Station ID"=Station_ID_Selector."B") -> ("error out"=w586:errorcluster)  [unwired: 7 in, 2 out]
              }
            }
          }
          frame Enabled {
          }
        }
        n165 = call "INTELLIFAUCET DO Control.vi"("VISA session"=w575, "HEWH MW100 Channel Numbers"=T4 "053", "Normally Open"=w572, "Error In"=w576) -> ("dup VISA session"=w574:refnum<visa-resource-name>, "error out"=w577:errorcluster)  [unwired: 10 in]
        n166 = case shown="Error .." w577 {
          selector: w577 -> [w589 _]
          tunnel: [w588 w592] -> w583
          tunnel: w582 -> [w587 w591]
          frame No Error {
            n167 = call-poly "Enqueue Message.vi"("error in (no error)"=w589, "Message"="Get_MW100_Data", "Message Queue"=w587) -> ("error out"=w588:errorcluster)  [unwired: 7 in, 1 out]
          }
          frame Error {
            n168 = call-poly "Enqueue Message.vi"("Message"="Connect_MW100", "Message Queue"=w591) -> ("error out"=w592:errorcluster)  [unwired: 8 in, 1 out]
          }
        }
      }
      frame "Inlet_Valve_C_MW100" {
        # "Check this one. Think its reversed."
        n169 = Variant To Data(error in=w604, type=T5 "ON" ("Input Valve"), Variant=w603) -> (data=w596:T5, error out=w600:errorcluster)
        n170 = disable-structure shown="Disabled" {
          frame Disabled {
            n171 = case shown="\"PRAT\"" {
              selector: _ -> [_ _]
              frame Default {
                n172 = call "Solenoid - Fill.vi"() -> ()  [unwired: 10 in, 2 out]
              }
              frame "PRAT" {
                n173 = call "HEWH PRAT Valves.vi"("Normally Closed Valve?"=TRUE, "Station ID"=Station_ID_Selector."C") -> ()  [unwired: 7 in, 3 out]
              }
            }
          }
          frame Enabled {
          }
        }
        n174 = call "INTELLIFAUCET DO Control.vi"("VISA session"=w599, "HEWH MW100 Channel Numbers"=T4 "057", "Normally Open"=w596, "Error In"=w600) -> ("dup VISA session"=w598:refnum<visa-resource-name>, "error out"=w601:errorcluster)  [unwired: 10 in]
        n175 = case shown="Error .." w601 {
          selector: w601 -> [w612 _]
          tunnel: [w611 w615] -> w607
          tunnel: w606 -> [w610 w614]
          frame No Error {
            n176 = call-poly "Enqueue Message.vi"("error in (no error)"=w612, "Message"="Get_MW100_Data", "Message Queue"=w610) -> ("error out"=w611:errorcluster)  [unwired: 7 in, 1 out]
          }
          frame Error {
            n177 = call-poly "Enqueue Message.vi"("Message"="Connect_MW100", "Message Queue"=w614) -> ("error out"=w615:errorcluster)  [unwired: 8 in, 1 out]
          }
        }
      }
      frame "Inlet_Valve_D_MW100" {
        # "Check this one. Think its reversed."
        n178 = Variant To Data(error in=w627, type=T5 "ON" ("Input Valve"), Variant=w626) -> (data=w619:T5, error out=w624:errorcluster)
        n179 = disable-structure shown="Disabled" {
          frame Disabled {
            n180 = case shown="\"PRAT\"" {
              selector: _ -> [_ _]
              frame Default {
                n181 = call "Solenoid - Fill.vi"() -> ()  [unwired: 10 in, 2 out]
              }
              frame "PRAT" {
                n182 = call "HEWH PRAT Valves.vi"("Normally Closed Valve?"=TRUE, "Station ID"=Station_ID_Selector."D") -> ()  [unwired: 7 in, 3 out]
              }
            }
          }
          frame Enabled {
          }
        }
        n183 = call "INTELLIFAUCET DO Control.vi"("VISA session"=w622, "HEWH MW100 Channel Numbers"=T4 "060", "Normally Open"=w619, "Error In"=w624) -> ("dup VISA session"=w621:refnum<visa-resource-name>, "error out"=w625:errorcluster)  [unwired: 10 in]
        n184 = case shown="Error .." w625 {
          selector: w625 -> [w635 _]
          tunnel: [w634 w638] -> w630
          tunnel: w629 -> [w633 w637]
          frame No Error {
            n185 = call-poly "Enqueue Message.vi"("error in (no error)"=w635, "Message"="Get_MW100_Data", "Message Queue"=w633) -> ("error out"=w634:errorcluster)  [unwired: 7 in, 1 out]
          }
          frame Error {
            n186 = call-poly "Enqueue Message.vi"("Message"="Connect_MW100", "Message Queue"=w637) -> ("error out"=w638:errorcluster)  [unwired: 8 in, 1 out]
          }
        }
      }
      frame "Drain_Valve_A_MW100" {
        n187 = Variant To Data(error in=w650, type=T7 "OFF" ("Normally Closed Valve"), Variant=w649) -> (data=w642:T7, error out=w645:errorcluster)
        n188 = disable-structure shown="Disabled" {
          frame Disabled {
            n189 = call "Solenoid - DRAIN.vi"() -> ()  [unwired: 10 in, 2 out]
          }
          frame Enabled {
          }
        }
        n190 = call "HEWH_Normally_Closed_Solenoid.vi"("VISA session"=w648, "HEWH MW100 Channel Numbers"=T4 "048", "Normally Closed"=w642, "Error In"=w645) -> ("dup VISA session"=w647:refnum<visa-resource-name>, "error out"=w644:errorcluster)  [unwired: 10 in]
        n191 = case shown="Error .." w644 {
          selector: w644 -> [w656 _]
          tunnel: [w655 w659] -> w653
          tunnel: w652 -> [w654 w658]
          frame No Error {
            n192 = call-poly "Enqueue Message.vi"("error in (no error)"=w656, "Message"="Get_MW100_Data", "Message Queue"=w654) -> ("error out"=w655:errorcluster)  [unwired: 7 in, 1 out]
          }
          frame Error {
            n193 = call-poly "Enqueue Message.vi"("Message"="Connect_MW100", "Message Queue"=w658) -> ("error out"=w659:errorcluster)  [unwired: 8 in, 1 out]
          }
        }
      }
      frame "Drain_Valve_B_MW100" {
        n194 = Variant To Data(error in=w671, type=T7 "OFF" ("Normally Closed Valve"), Variant=w670) -> (data=w663:T7, error out=w669:errorcluster)
        n195 = disable-structure shown="Disabled" {
          frame Disabled {
            n196 = call "Solenoid - DRAIN.vi"() -> ()  [unwired: 10 in, 2 out]
          }
          frame Enabled {
          }
        }
        n197 = call "HEWH_Normally_Closed_Solenoid.vi"("VISA session"=w666, "HEWH MW100 Channel Numbers"=T4 "051", "Normally Closed"=w663, "Error In"=w669) -> ("dup VISA session"=w665:refnum<visa-resource-name>, "error out"=w668:errorcluster)  [unwired: 10 in]
        n198 = case shown="Error .." w668 {
          selector: w668 -> [w677 _]
          tunnel: [w676 w680] -> w674
          tunnel: w673 -> [w675 w679]
          frame No Error {
            n199 = call-poly "Enqueue Message.vi"("error in (no error)"=w677, "Message"="Get_MW100_Data", "Message Queue"=w675) -> ("error out"=w676:errorcluster)  [unwired: 7 in, 1 out]
          }
          frame Error {
            n200 = call-poly "Enqueue Message.vi"("Message"="Connect_MW100", "Message Queue"=w679) -> ("error out"=w680:errorcluster)  [unwired: 8 in, 1 out]
          }
        }
      }
      frame "Drain_Valve_C_MW100" {
        n201 = Variant To Data(error in=w692, type=T7 "OFF" ("Normally Closed Valve"), Variant=w691) -> (data=w684:T7, error out=w690:errorcluster)
        n202 = disable-structure shown="Disabled" {
          frame Disabled {
            n203 = call "Solenoid - DRAIN.vi"() -> ()  [unwired: 10 in, 2 out]
          }
          frame Enabled {
          }
        }
        n204 = call "HEWH_Normally_Closed_Solenoid.vi"("VISA session"=w688, "HEWH MW100 Channel Numbers"=T4 "054", "Normally Closed"=w684, "Error In"=w690) -> ("dup VISA session"=w687:refnum<visa-resource-name>, "error out"=w689:errorcluster)  [unwired: 10 in]
        n205 = case shown="Error .." w689 {
          selector: w689 -> [w698 _]
          tunnel: [w697 w701] -> w695
          tunnel: w694 -> [w696 w700]
          frame No Error {
            n206 = call-poly "Enqueue Message.vi"("error in (no error)"=w698, "Message"="Get_MW100_Data", "Message Queue"=w696) -> ("error out"=w697:errorcluster)  [unwired: 7 in, 1 out]
          }
          frame Error {
            n207 = call-poly "Enqueue Message.vi"("Message"="Connect_MW100", "Message Queue"=w700) -> ("error out"=w701:errorcluster)  [unwired: 8 in, 1 out]
          }
        }
      }
      frame "Drain_Valve_D_MW100" {
        n208 = Variant To Data(error in=w713, type=T7 "OFF" ("Normally Closed Valve"), Variant=w712) -> (data=w705:T7, error out=w710:errorcluster)
        n209 = disable-structure shown="Disabled" {
          frame Disabled {
            n210 = call "Solenoid - DRAIN.vi"() -> ()  [unwired: 10 in, 2 out]
          }
          frame Enabled {
          }
        }
        n211 = call "HEWH_Normally_Closed_Solenoid.vi"("VISA session"=w709, "HEWH MW100 Channel Numbers"=T4 "058", "Normally Closed"=w705, "Error In"=w710) -> ("dup VISA session"=w708:refnum<visa-resource-name>, "error out"=w711:errorcluster)  [unwired: 10 in]
        n212 = case shown="Error .." w711 {
          selector: w711 -> [w719 _]
          tunnel: [w718 w722] -> w716
          tunnel: w715 -> [w717 w721]
          frame No Error {
            n213 = call-poly "Enqueue Message.vi"("error in (no error)"=w719, "Message"="Get_MW100_Data", "Message Queue"=w717) -> ("error out"=w718:errorcluster)  [unwired: 7 in, 1 out]
          }
          frame Error {
            n214 = call-poly "Enqueue Message.vi"("Message"="Connect_MW100", "Message Queue"=w721) -> ("error out"=w722:errorcluster)  [unwired: 8 in, 1 out]
          }
        }
      }
      frame "Outlet_Valve_A_MW100" {
        n215 = Variant To Data(error in=w734, type=T5 "ON" ("Input Valve"), Variant=w733) -> (data=w726:T5, error out=w732:errorcluster)
        n216 = disable-structure shown="Disabled" {
          frame Disabled {
            n217 = call "HEWH Solenoid Output Set.vi"() -> ()  [unwired: 10 in, 2 out]
          }
          frame Enabled {
          }
        }
        n218 = call "INTELLIFAUCET DO Control.vi"("VISA session"=w729, "HEWH MW100 Channel Numbers"=T4 "049", "Normally Open"=w726, "Error In"=w732) -> ("dup VISA session"=w728:refnum<visa-resource-name>, "error out"=w731:errorcluster)  [unwired: 10 in]
        n219 = case shown="Error .." w731 {
          selector: w731 -> [w740 _]
          tunnel: [w739 w743] -> w737
          tunnel: w736 -> [w738 w742]
          frame No Error {
            n220 = call-poly "Enqueue Message.vi"("error in (no error)"=w740, "Message"="Get_MW100_Data", "Message Queue"=w738) -> ("error out"=w739:errorcluster)  [unwired: 7 in, 1 out]
          }
          frame Error {
            n221 = call-poly "Enqueue Message.vi"("Message"="Connect_MW100", "Message Queue"=w742) -> ("error out"=w743:errorcluster)  [unwired: 8 in, 1 out]
          }
        }
      }
      frame "Outlet_Valve_B_MW100" {
        n222 = Variant To Data(error in=w755, type=T5 "ON" ("Input Valve"), Variant=w754) -> (data=w747:T5, error out=w753:errorcluster)
        n223 = disable-structure shown="Disabled" {
          frame Disabled {
            n224 = call "HEWH Solenoid Output Set.vi"() -> ()  [unwired: 10 in, 2 out]
          }
          frame Enabled {
          }
        }
        n225 = call "INTELLIFAUCET DO Control.vi"("VISA session"=w751, "HEWH MW100 Channel Numbers"=T4 "052", "Normally Open"=w747, "Error In"=w753) -> ("dup VISA session"=w750:refnum<visa-resource-name>, "error out"=w752:errorcluster)  [unwired: 10 in]
        n226 = case shown="Error .." w752 {
          selector: w752 -> [w761 _]
          tunnel: [w760 w764] -> w758
          tunnel: w757 -> [w759 w763]
          frame No Error {
            n227 = call-poly "Enqueue Message.vi"("error in (no error)"=w761, "Message"="Get_MW100_Data", "Message Queue"=w759) -> ("error out"=w760:errorcluster)  [unwired: 7 in, 1 out]
          }
          frame Error {
            n228 = call-poly "Enqueue Message.vi"("Message"="Connect_MW100", "Message Queue"=w763) -> ("error out"=w764:errorcluster)  [unwired: 8 in, 1 out]
          }
        }
      }
      frame "Outlet_Valve_C_MW100" {
        n229 = Variant To Data(error in=w776, type=T5 "ON" ("Input Valve"), Variant=w775) -> (data=w768:T5, error out=w773:errorcluster)
        n230 = disable-structure shown="Disabled" {
          frame Disabled {
            n231 = call "HEWH Solenoid Output Set.vi"() -> ()  [unwired: 10 in, 2 out]
          }
          frame Enabled {
          }
        }
        n232 = call "INTELLIFAUCET DO Control.vi"("VISA session"=w772, "HEWH MW100 Channel Numbers"=T4 "055", "Normally Open"=w768, "Error In"=w773) -> ("dup VISA session"=w771:refnum<visa-resource-name>, "error out"=w774:errorcluster)  [unwired: 10 in]
        n233 = case shown="Error .." w774 {
          selector: w774 -> [w782 _]
          tunnel: [w781 w785] -> w779
          tunnel: w778 -> [w780 w784]
          frame No Error {
            n234 = call-poly "Enqueue Message.vi"("error in (no error)"=w782, "Message"="Get_MW100_Data", "Message Queue"=w780) -> ("error out"=w781:errorcluster)  [unwired: 7 in, 1 out]
          }
          frame Error {
            n235 = call-poly "Enqueue Message.vi"("Message"="Connect_MW100", "Message Queue"=w784) -> ("error out"=w785:errorcluster)  [unwired: 8 in, 1 out]
          }
        }
      }
      frame "Outlet_Valve_D_MW100" {
        n236 = Variant To Data(error in=w797, type=T5 "ON" ("Input Valve"), Variant=w796) -> (data=w789:T5, error out=w794:errorcluster)
        n237 = disable-structure shown="Disabled" {
          frame Disabled {
            n238 = call "HEWH Solenoid Output Set.vi"() -> ()  [unwired: 10 in, 2 out]
          }
          frame Enabled {
          }
        }
        n239 = call "INTELLIFAUCET DO Control.vi"("VISA session"=w792, "HEWH MW100 Channel Numbers"=T4 "059", "Normally Open"=w789, "Error In"=w794) -> ("dup VISA session"=w791:refnum<visa-resource-name>, "error out"=w795:errorcluster)  [unwired: 10 in]
        n240 = case shown="Error .." w795 {
          selector: w795 -> [w803 _]
          tunnel: [w802 w806] -> w800
          tunnel: w799 -> [w801 w805]
          frame No Error {
            n241 = call-poly "Enqueue Message.vi"("error in (no error)"=w803, "Message"="Get_MW100_Data", "Message Queue"=w801) -> ("error out"=w802:errorcluster)  [unwired: 7 in, 1 out]
          }
          frame Error {
            n242 = call-poly "Enqueue Message.vi"("Message"="Connect_MW100", "Message Queue"=w805) -> ("error out"=w806:errorcluster)  [unwired: 8 in, 1 out]
          }
        }
      }
      frame "---------- Intellifaucet Control ----------" {
      }
      frame "Start_Intellifaucet_MW100" {
        n243 = disable-structure shown="Disabled" {
          frame Disabled {
            (unwired) "Start Intellifaucet\nAdjust Flow\nAdjust Temp" ("State(s) in Front (\"\")")
            n244 = call "INTELLIFAUCET Driver.vi"("Mode"=INTELLIFAUCET_Set_Mode."Start Flow") -> ()  [unwired: 12 in, 3 out]
          }
          frame Enabled {
          }
        }
        n245 = call "INTELLIFAUCET Start Stop.vi"("Start?"=TRUE, "error in (no error)"=w818, "VISA Refnum in"=w819) -> ("error out"=w815:errorcluster, "VISA Refnum out"=w816:refnum<visa-resource-name>)  [unwired: 7 in]
        n246 = case shown="Error .." w815 {
          selector: w815 -> [w826 _]
          tunnel: [w825 w829] -> w822
          tunnel: w821 -> [w824 w828]
          frame No Error {
            n247 = call-poly "Enqueue Message.vi"("error in (no error)"=w826, "Message"="Get_MW100_Data", "Message Queue"=w824) -> ("error out"=w825:errorcluster)  [unwired: 7 in, 1 out]
          }
          frame Error {
            n248 = call-poly "Enqueue Message.vi"("Message"="Connect_MW100", "Message Queue"=w828) -> ("error out"=w829:errorcluster)  [unwired: 8 in, 1 out]
          }
        }
      }
      frame "Stop_Intellifaucet_MW100" {
        n249 = disable-structure shown="Disabled" {
          frame Disabled {
            n250 = call "INTELLIFAUCET Driver.vi"("Mode"=INTELLIFAUCET_Set_Mode."Stop Flow") -> ()  [unwired: 12 in, 3 out]
          }
          frame Enabled {
          }
        }
        n251 = call "INTELLIFAUCET Start Stop.vi"("Start?"=FALSE, "error in (no error)"=w835, "VISA Refnum in"=w833) -> ("error out"=w834:errorcluster, "VISA Refnum out"=w832:refnum<visa-resource-name>)  [unwired: 7 in]
        n252 = case shown="No Error" w834 {
          selector: w834 -> [w844 _]
          tunnel: [w843 w847] -> w840
          tunnel: w839 -> [w842 w846]
          frame No Error {
            n253 = call-poly "Enqueue Message.vi"("error in (no error)"=w844, "Message"="Get_MW100_Data", "Message Queue"=w842) -> ("error out"=w843:errorcluster)  [unwired: 7 in, 1 out]
          }
          frame Error {
            n254 = call-poly "Enqueue Message.vi"("Message"="Connect_MW100", "Message Queue"=w846) -> ("error out"=w847:errorcluster)  [unwired: 8 in, 1 out]
          }
        }
      }
      frame "Adjust_Temp_Intellifaucet_MW100" {
        n255 = Variant To Data(error in=w861, type=0.0, Variant=w860) -> (data=w858:dbl, error out=w856:errorcluster)
        n256 = call "HEWH Intellifaucet Temp Equation.vi"("Error In"=w856, "Temp Target (F)"=w858) -> ("Error Out"=w854:errorcluster, "Temp uA"=w850:i32)  [unwired: 7 in, 1 out]
        n257 = disable-structure shown="Disabled" {
          frame Disabled {
            # "Operate this on Approx Values\n(Dont wire the 2D Array)"
            n258 = call "UTILITY Delay mS.vi"("milliseconds to wait"=u32 50) -> ()  [unwired: 14 in, 1 out]
            n259 = call "INTELLIFAUCET Driver.vi"("Mode"=INTELLIFAUCET_Set_Mode."Adjust Temp", "Use General Conversion"=TRUE) -> ()  [unwired: 11 in, 3 out]
          }
          frame Enabled {
          }
        }
        n260 = call "INTELLIFAUCET Temp Flow.vi"("Temperature (T), Flow (F)"=TRUE, "error in (no error)"=w854, "uA Output"=w850, "VISA Refnum in"=w851) -> ("error out"=w853:errorcluster, "VISA Refnum out"=w852:refnum<visa-resource-name>)  [unwired: 6 in]
        n261 = case shown="Error .." w853 {
          selector: w853 -> [w870 _]
          tunnel: [w869 w873] -> w864
          tunnel: w863 -> [w868 w872]
          frame No Error {
            n262 = call-poly "Enqueue Message.vi"("error in (no error)"=w870, "Message"="Get_MW100_Data", "Message Queue"=w868) -> ("error out"=w869:errorcluster)  [unwired: 7 in, 1 out]
          }
          frame Error {
            n263 = call-poly "Enqueue Message.vi"("Message"="Connect_MW100", "Message Queue"=w872) -> ("error out"=w873:errorcluster)  [unwired: 8 in, 1 out]
          }
        }
      }
      frame "Adjust_Flow_Intellifaucet_MW100" {
        n264 = Variant To Data(error in=w888, type=0.0, Variant=w887) -> (data=w882:dbl, error out=w877:errorcluster)
        n265 = call "INTELLIFAUCET Linear Interpolation GPMtouA.vi"("Error In"=w877, "Flow Value"=w882) -> ("Error Out"=w884:errorcluster, "uA Output"=w881:i32)  [unwired: 8 in]
        n266 = disable-structure shown="Disabled" {
          frame Disabled {
            n267 = call "UTILITY Delay mS.vi"("milliseconds to wait"=u32 50) -> ()  [unwired: 14 in, 1 out]
            n268 = call "INTELLIFAUCET Driver.vi"("Mode"=INTELLIFAUCET_Set_Mode."Adjust Flow", "Use General Conversion"=TRUE) -> ()  [unwired: 11 in, 3 out]
          }
          frame Enabled {
          }
        }
        n269 = call "INTELLIFAUCET Temp Flow.vi"("Temperature (T), Flow (F)"=FALSE, "error in (no error)"=w884, "uA Output"=w881, "VISA Refnum in"=w883) -> ("error out"=w878:errorcluster, "VISA Refnum out"=w880:refnum<visa-resource-name>)  [unwired: 6 in]
        n270 = case shown="Error .." w878 {
          selector: w878 -> [w896 _]
          tunnel: [w895 w899] -> w890
          tunnel: w889 -> [w894 w898]
          frame No Error {
            n271 = call-poly "Enqueue Message.vi"("error in (no error)"=w896, "Message"="Get_MW100_Data", "Message Queue"=w894) -> ("error out"=w895:errorcluster)  [unwired: 7 in, 1 out]
          }
          frame Error {
            n272 = call-poly "Enqueue Message.vi"("Message"="Connect_MW100", "Message Queue"=w898) -> ("error out"=w899:errorcluster)  [unwired: 8 in, 1 out]
          }
        }
      }
      frame "---------- Proportion Valve Control ----------" {
      }
      frame "Adjust_Prop_Valve_MW100" {
        n273 = Variant To Data(error in=w923, type=0.0, Variant=w922) -> (data=w917:dbl, error out=w919:errorcluster)
        n274 = case shown="False" "Use Micro Amp Set" {
          tunnel: w919 -> [w932 w935]
          tunnel: [w931 w935] -> w916
          tunnel: [w927 w936] -> w911
          tunnel: w917 -> [w926 w936]
          frame False {
            n275 = call "UTILITY Fuzzy Logic Scale.vi"("Convert to MicroAmp (T), Standard Output (F)"=TRUE, "Error In"=w932, "input variable"=w926, "output range"=cluster{"output high":dbl, "output low":dbl} {"output high"=100.0, "output low"=0.0}) -> ("Error Out"=w931:errorcluster, "MicroAmp"=w928:dbl)  [unwired: 6 in]
            n276 = In Range and Coerce(upper limit=20000.0, x=w928, lower limit=4000.0) -> (coerced(x)=w927:dbl)  [unwired: 1 out]
          }
          frame True {
          }
        }
        n277 = disable-structure shown="Disabled" {
          frame Disabled {
            n278 = call "UTILITY Delay mS.vi"("milliseconds to wait"=u32 100) -> ()  [unwired: 14 in, 1 out]
            n279 = call "PROPORTIONING VALVE MicroAmp Set.vi"("milliseconds to wait"=u32 100, "Use Micro Amp Set"=FALSE) -> ()  [unwired: 8 in, 2 out]
          }
          frame Enabled {
          }
        }
        n280 = call "YKMW100 Clear Output Buffer.vi"("VISA session"=w915, "error in (no error)"=w916) -> ("dup VISA session"=w913:refnum<visa-resource-name>, "error out"=w914:errorcluster)  [unwired: 12 in]
        n281 = To Long Integer(number=w911) -> (32bit integer=w910:i32)
        n282 = call "YKMW100 Output AO.vi"("VISA session"=w913, "Channel String (001)"=T4 "002" ("HEWH MW100 Channel Numbers"), "Output Value (0)"=w910, "error in (no error)"=w914) -> ("dup VISA session"=w909:refnum<visa-resource-name>, "error out"=w907:errorcluster)  [unwired: 10 in]
        n283 = case shown="Error .." w907 {
          selector: w907 -> [w942 _]
          tunnel: [w941 w945] -> w925
          tunnel: w924 -> [w940 w944]
          frame No Error {
            n284 = call-poly "Enqueue Message.vi"("error in (no error)"=w942, "Message"="Get_MW100_Data", "Message Queue"=w940) -> ("error out"=w941:errorcluster)  [unwired: 7 in, 1 out]
          }
          frame Error {
            n285 = call-poly "Enqueue Message.vi"("Message"="Connect_MW100", "Message Queue"=w944) -> ("error out"=w945:errorcluster)  [unwired: 8 in, 1 out]
          }
        }
      }
    }
    n286 = case shown="True" "Debug" {
      tunnel: w80 -> [_ w95]
      tunnel: w79 -> [w92 w94]
      tunnel: [w92 w93] -> w78
      frame False {
      }
      frame True {
        n287 = Build Array (concatenate)(w94, w95) -> (w93:string[])
        "Debug" <- w93
      }
    }
    n288 = Wait Until Next ms Multiple(millisecond multiple=w72) -> ()  [unwired: 1 out]
    n289 = call "Error Handler - Message Handling Loop.vi"("error in (no error)"=w85, "Message Queue"=w87) -> ("dup error in"=w86:errorcluster)  [unwired: 8 in, 1 out]
    "Loop Count" <- w73
  }
  "error out" <- w3
